vi "PLC_comm.vi"() -> ()   [LabVIEW 2017]
uses:
  <vilib>/DATA AHEAD/SP7/typedefs/PLC Type.ctl
  <vilib>/Utility/error.llb/DialogType.ctl
  <vilib>/addons/database/Connection.llb/DB Tools Open Connec (String).vi
  <vilib>/DATA AHEAD/SP7/functions/write/write Dint array.vi
  Global/Global 1.vi
  Global/DATA LOG.vi
  <vilib>/DATA AHEAD/SP7/functions/write/writeString.vi
  <vilib>/DATA AHEAD/SP7/functions/read/read Dint array.vi
  <vilib>/DATA AHEAD/SP7/functions/read/read real array.vi
  <vilib>/DATA AHEAD/SP7/functions/read/read String.vi
  <vilib>/addons/database/NI_Database_API.lvlib
  <vilib>/DATA AHEAD/SP7/SP7.lvlib
panel:
  out "error out 4":errorcluster
  out "error out 3":errorcluster
  out "error out 2":errorcluster
  out "IP1 8":string
  out "PLC 8":bool
  out "IP1 7":string
  out "PLC 7":bool
  out "IP1 6":string
  out "PLC 6":bool
  out "IP1 5":string
  out "PLC 5":bool
  out "PLC 4":bool
  out "PLC 3":bool
  out "PLC 2":bool
  out "PLC 1":bool
  out "IP1 4":string
  out "IP1 3":string
  out "IP1 2":string
  out "IP1":string
  in  "stop":bool
  out "error out":errorcluster
  in  "error in (no error)":errorcluster
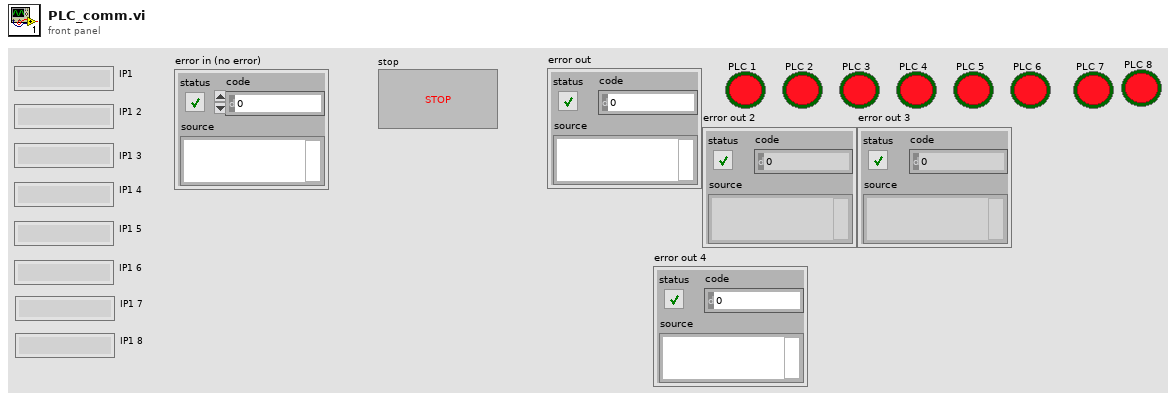
[diagram p1: front panel]
types:
  T1 = typedef "SP7.lvlib/PLC Type.ctl" = enum16{"S7 200", "S7 300/400", "S7 1200", "S7 1500", "LOGO!8"}
  T2 = typedef "DialogType.ctl" = u16
  T3 = typedef "NI_Database_API.lvlib/Conn ObjectReference.ctl" = refnum<k1>
  T4 = typedef "SP7.lvlib/S7 Connection.ctl" = cluster{"TCP Connection Ref":refnum<k5>, "IP address":string, "timeout ms":i32, "Connected?":bool, "PLC Type":T1, "Rack S7 400":u8, "Slot S7 400":u8, "PDU Size":u16, "connection semaphore":T5}
  T5 = typedef "Semaphore RefNum" = refnum<k1>
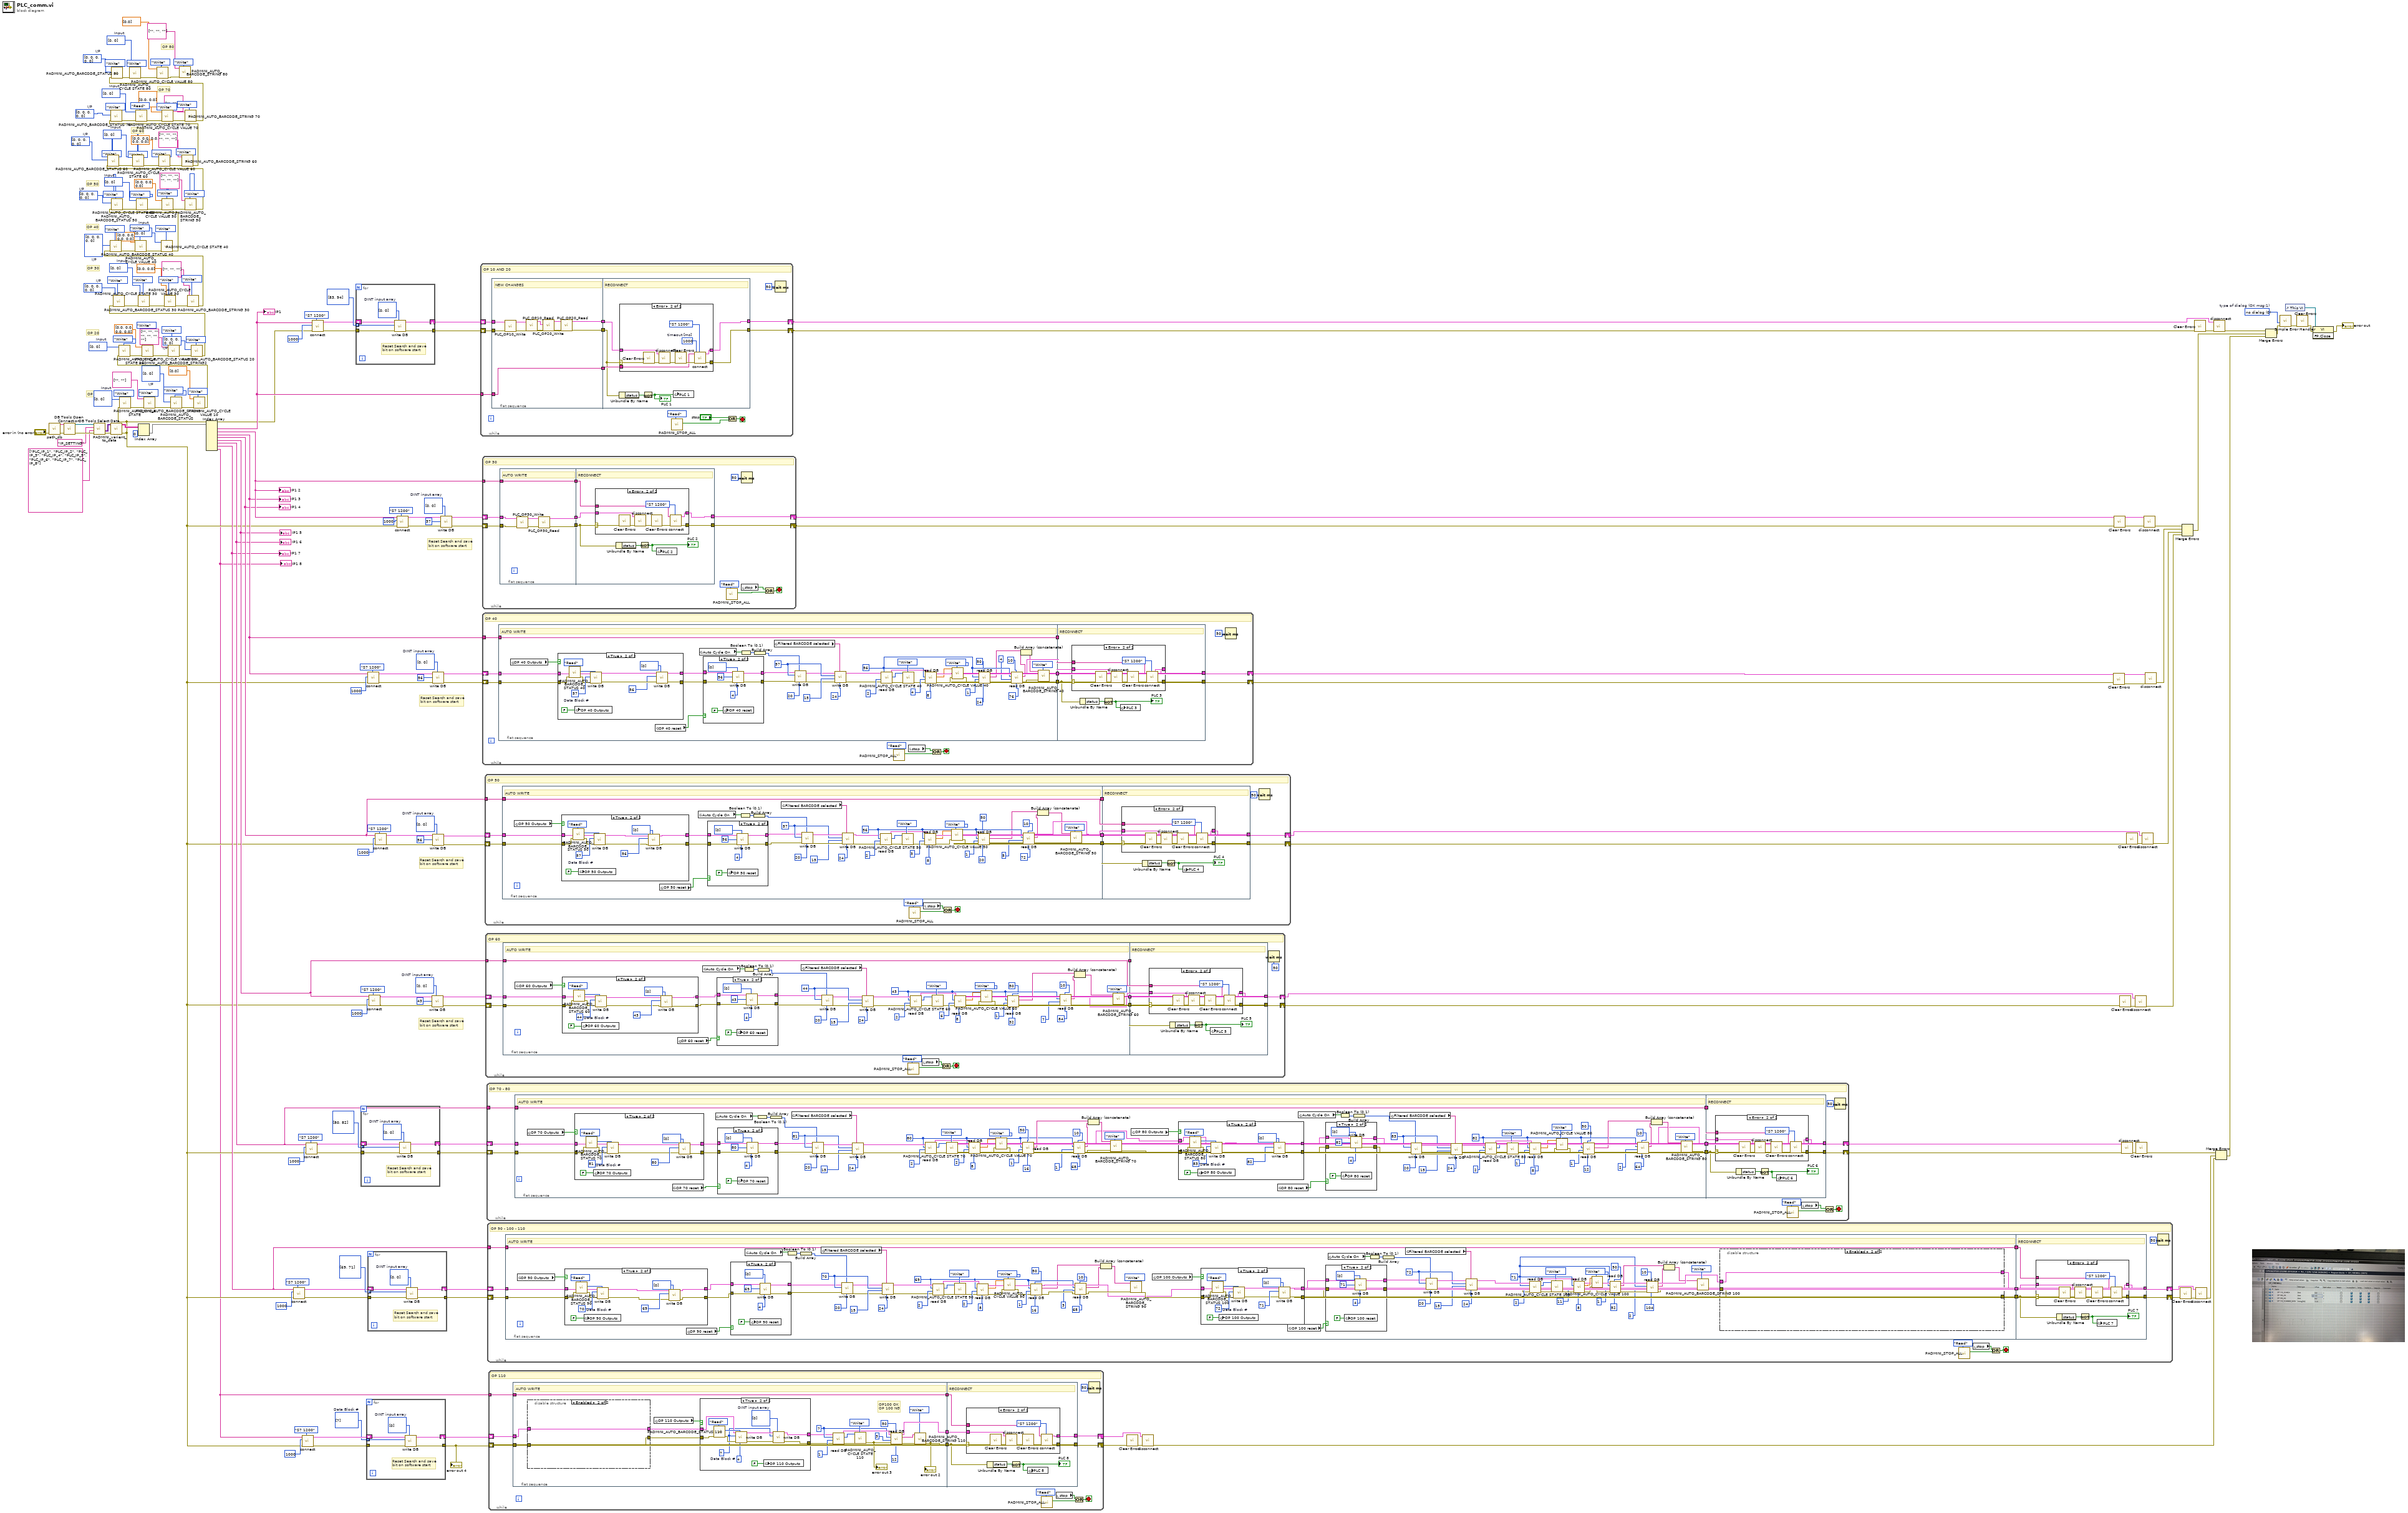
[diagram p0: block diagram]
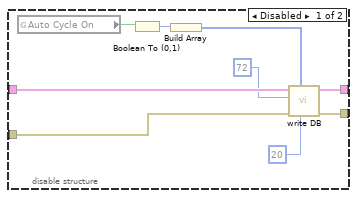
[diagram p2: hidden frame]
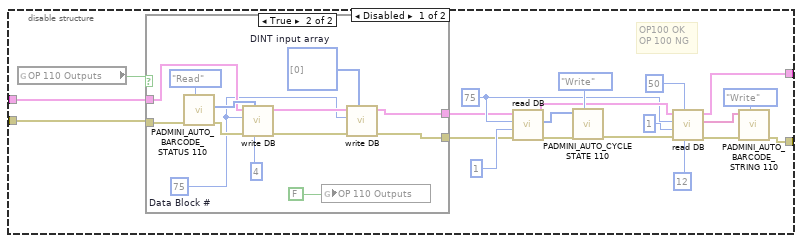
[diagram p5: hidden frame]
diagram:
  w6 = u16[] [7]  # Data Block #
  w28 = i32[] [0, 0]  # DINT input array
  w35 = i32[] [0, 0]  # DINT input array
  w40 = i32[] [0, 0]  # DINT input array
  w52 = i32[] [0, 0]  # DINT input array
  w53 = T2 0 items=["no dialog", "OK message", "continue or stop message", "OK message + warnings", "continue/stop + warnings"]  # type of dialog (OK msg:1)
  w55 = i32[] [0, 0, 0, 0, 0]  # I/P
  w56 = i32[] [0, 0]  # Input
  w58 = i32[] [0, 0]  # Input
  w59 = i32[] [0, 0]  # Input
  w61 = i32[] [0, 0]  # Input
  w57 = i32[] [0, 0, 0, 0, 0]  # I/P
  w60 = i32[] [0, 0, 0, 0, 0]  # I/P
  w62 = i32[] [0, 0, 0, 0, 0]  # I/P
  w63 = i32[] [0, 0, 0, 0, 0]  # I/P
  w64 = i32[] [0, 0]  # Input
  w65 = i32[] [0, 0]  # Input
  w66 = i32[] [0, 0, 0, 0, 0]  # I/P
  w67 = i32[] [0, 0, 0, 0, 0]  # I/P
  w68 = i32[] [0, 0]  # Input
  w69 = i32[] [0, 0]  # I/P
  w70 = i32[] [0, 0]  # Input
  # "Reset Search and save \nbit on software start"
  # "Reset Search and save \nbit on software start"
  # "Reset Search and save \nbit on software start"
  # "Reset Search and save \nbit on software start"
  # "OP 80"
  # "OP 70"
  # "OP 60"
  # "OP 50"
  # "OP 40"
  # "OP 30"
  # "OP 20"
  # "OP 10"
  n1 = call "path_db.vi"("error in"="error in (no error)") -> ("error out"=w208:errorcluster, "resulting string"=w213:string)  [unwired: 9 in]
  n2 = call-poly <vilib>:"DB Tools Open Connection.vi"("error in (no error)"=w208, "connection information"=w213) -> ("error out"=w212:errorcluster, "connection reference"=w211:T3)  [unwired: 6 in]
  n3 = call <vilib>:"DB Tools Select Data.vi"("error in (no error)"=w212, "columns"=string[] ["PLC_IP_1", "PLC_IP_2", "PLC_IP_3", "PLC_IP_4", "PLC_IP_5", "PLC_IP_6", "PLC_IP_7", "PLC_IP_8"], "table"="IP_SETTING", "connection reference"=w211) -> ("error out"=w210:errorcluster, "data"=w209:variant[][])  [unwired: 2 in, 1 out]
  n4 = call "PADMINI_varient_to_data.vi"("error in (no error)"=w210, "data"=w209) -> ("error out"=w7:errorcluster, "Array"=w204:string[][])  [unwired: 8 in]
  n5 = call "PADMINI_AUTO_CYCLE STATE.vi"("Enum"=enum16{"Read", "Write"}."Write", "error in (no error)"=w7, "Input"=w70) -> ("error out"=w192:errorcluster)  [unwired: 7 in, 1 out]
  n6 = Index Array(array=w204, index (row)=0) -> (element=w203:string[])  [unwired: 1 in]
  n7 = call "PADMINI_AUTO_BARCODE_STRING.vi"("Enum"=enum16{"Read", "Write"}."Write", "error in (no error)"=w192, "Input"=string[] ["", ""]) -> ("error out"=w189:errorcluster)  [unwired: 7 in, 1 out]
  n8 = call "PADMINI_AUTO_BARCODE_STATUS.vi"("Enum"=enum16{"Read", "Write"}."Write", "error in (no error)"=w189, "I/P"=w69) -> ("error out"=w187:errorcluster)  [unwired: 7 in, 1 out]
  n9 = call "PADMINI_AUTO_CYCLE VALUE 10.vi"("Enum"=enum16{"Read", "Write"}."Write", "error in (no error)"=w187, "Input"=dbl[] [0.0]) -> ("error out"=w181:errorcluster)  [unwired: 7 in, 1 out]
  n10 = call "PADMINI_AUTO_CYCLE STATE 20.vi"("Enum"=enum16{"Read", "Write"}."Write", "error in (no error)"=w181, "Input"=w56) -> ("error out"=w179:errorcluster)  [unwired: 7 in, 1 out]
  n11 = call "PADMINI_AUTO_CYCLE VALUE 20.vi"("Enum"=enum16{"Read", "Write"}."Write", "error in (no error)"=w179, "Input"=dbl[] [0.0, 0.0, 0.0, 0.0]) -> ("error out"=w175:errorcluster)  [unwired: 7 in, 1 out]
  n12 = call "PADMINI_AUTO_BARCODE_STRING2.vi"("Enum"=enum16{"Read", "Write"}."Write", "error in (no error)"=w175, "Input"=string[] ["", "", "", "", "", "", ""]) -> ("error out"=w173:errorcluster)  [unwired: 7 in, 1 out]
  n13 = call "PADMINI_AUTO_BARCODE_STATUS 20.vi"("Enum"=enum16{"Read", "Write"}."Write", "error in (no error)"=w173, "I/P"=w55) -> ("error out"=w169:errorcluster)  [unwired: 7 in, 1 out]
  n14 = call "PADMINI_AUTO_BARCODE_STATUS 30.vi"("Enum"=enum16{"Read", "Write"}."Write", "error in (no error)"=w169, "I/P"=w57) -> ("error out"=w166:errorcluster)  [unwired: 7 in, 1 out]
  n15 = call "PADMINI_AUTO_CYCLE STATE 30.vi"("Enum"=enum16{"Read", "Write"}."Write", "error in (no error)"=w166, "Input"=w58) -> ("error out"=w165:errorcluster)  [unwired: 7 in, 1 out]
  n16 = call "PADMINI_AUTO_CYCLE VALUE 30.vi"("Enum"=enum16{"Read", "Write"}."Write", "error in (no error)"=w165, "Input"=dbl[] [0.0, 0.0]) -> ("error out"=w162:errorcluster)  [unwired: 7 in, 1 out]
  n17 = call "PADMINI_AUTO_BARCODE_STRING 30.vi"("Enum"=enum16{"Read", "Write"}."Write", "error in (no error)"=w162, "Input"=string[] ["", "", ""]) -> ("error out"=w143:errorcluster)  [unwired: 7 in, 1 out]
  n18 = call "PADMINI_AUTO_BARCODE_STATUS 40.vi"("Enum"=enum16{"Read", "Write"}."Write", "error in (no error)"=w143, "I/P"=w60) -> ("error out"=w142:errorcluster)  [unwired: 7 in, 1 out]
  n19 = call "PADMINI_AUTO_CYCLE VALUE 40.vi"("Enum"=enum16{"Read", "Write"}."Write", "error in (no error)"=w142, "Input"=dbl[] [0.0, 0.0, 0.0, 0.0]) -> ("error out"=w141:errorcluster)  [unwired: 7 in, 1 out]
  n20 = call "PADMINI_AUTO_CYCLE STATE 40.vi"("Enum"=enum16{"Read", "Write"}."Write", "error in (no error)"=w141, "Input"=w59) -> ("error out"=w140:errorcluster)  [unwired: 7 in, 1 out]
  n21 = call "PADMINI_AUTO_BARCODE_STATUS 50.vi"("Enum"=enum16{"Read", "Write"}."Write", "error in (no error)"=w140, "I/P"=w62) -> ("error out"=w127:errorcluster)  [unwired: 7 in, 1 out]
  n22 = call "PADMINI_AUTO_CYCLE STATE 50.vi"("Enum"=enum16{"Read", "Write"}."Write", "error in (no error)"=w127, "Input"=w61) -> ("error out"=w131:errorcluster)  [unwired: 7 in, 1 out]
  n23 = call "PADMINI_AUTO_CYCLE VALUE 50.vi"("Enum"=enum16{"Read", "Write"}."Write", "error in (no error)"=w131, "Input"=dbl[] [0.0, 0.0, 0.0]) -> ("error out"=w128:errorcluster)  [unwired: 7 in, 1 out]
  n24 = call "PADMINI_AUTO_BARCODE_STRING 50.vi"("Enum"=enum16{"Read", "Write"}."Write", "error in (no error)"=w128, "Input"=string[] ["", "", "", "", "", ""]) -> ("error out"=w106:errorcluster)  [unwired: 7 in, 1 out]
  n25 = call "PADMINI_AUTO_BARCODE_STATUS 60.vi"("Enum"=enum16{"Read", "Write"}."Write", "error in (no error)"=w106, "I/P"=w63) -> ("error out"=w110:errorcluster)  [unwired: 7 in, 1 out]
  n26 = call "PADMINI_AUTO_CYCLE STATE 60.vi"("Enum"=enum16{"Read", "Write"}."Write", "error in (no error)"=w110, "Input"=w64) -> ("error out"=w112:errorcluster)  [unwired: 7 in, 1 out]
  n27 = call "PADMINI_AUTO_CYCLE VALUE 60.vi"("Enum"=enum16{"Read", "Write"}."Write", "error in (no error)"=w112, "Input"=dbl[] [0.0, 0.0, 0.0, 0.0, 0.0]) -> ("error out"=w115:errorcluster)  [unwired: 7 in, 1 out]
  n28 = call "PADMINI_AUTO_BARCODE_STRING 60.vi"("Enum"=enum16{"Read", "Write"}."Write", "error in (no error)"=w115, "Input"=string[] ["", "", "", "", "", ""]) -> ("error out"=w84:errorcluster)  [unwired: 7 in, 1 out]
  n29 = call "PADMINI_AUTO_BARCODE_STATUS 70.vi"("Enum"=enum16{"Read", "Write"}."Write", "error in (no error)"=w84, "I/P"=w66) -> ("error out"=w87:errorcluster)  [unwired: 7 in, 1 out]
  n30 = call "PADMINI_AUTO_CYCLE STATE 70.vi"("Enum"=enum16{"Read", "Write"}."Read", "error in (no error)"=w87, "Input"=w65) -> ("error out"=w99:errorcluster)  [unwired: 7 in, 1 out]
  n31 = call "PADMINI_AUTO_CYCLE VALUE 70.vi"("Enum"=enum16{"Read", "Write"}."Write", "error in (no error)"=w99, "Input"=dbl[] [0.0, 0.0]) -> ("error out"=w96:errorcluster)  [unwired: 7 in, 1 out]
  n32 = call "PADMINI_AUTO_BARCODE_STRING 70.vi"("Enum"=enum16{"Read", "Write"}."Write", "error in (no error)"=w96, "Input"=string[] ["", ""]) -> ("error out"=w81:errorcluster)  [unwired: 7 in, 1 out]
  n33 = call "PADMINI_AUTO_BARCODE_STATUS 80.vi"("Enum"=enum16{"Read", "Write"}."Write", "error in (no error)"=w81, "I/P"=w67) -> ("error out"=w88:errorcluster)  [unwired: 7 in, 1 out]
  n34 = call "PADMINI_AUTO_CYCLE STATE 80.vi"("Enum"=enum16{"Read", "Write"}."Write", "error in (no error)"=w88, "Input"=w68) -> ("error out"=w92:errorcluster)  [unwired: 7 in, 1 out]
  n35 = call "PADMINI_AUTO_CYCLE VALUE 80.vi"("Enum"=enum16{"Read", "Write"}."Write", "error in (no error)"=w92, "Input"=sgl[] [0.0]) -> ("error out"=w95:errorcluster)  [unwired: 7 in, 1 out]
  n36 = call "PADMINI_AUTO_BARCODE_STRING 80.vi"("Enum"=enum16{"Read", "Write"}."Write", "error in (no error)"=w95, "Input"=string[] ["", "", ""]) -> ()  [unwired: 7 in, 2 out]
  n37 = Index Array(array=w203) -> (element #1=w156:string, element #2=w157:string, element #3=w153:string, element #4=w133:string, element #5=w118:string, element #6=w78:string, element #7=w77:string, element #8=w5:string)  [unwired: 8 in]
  "IP1" <- w156
  "IP1 2" <- w157
  "IP1 3" <- w153
  "IP1 4" <- w133
  "IP1 5" <- w118
  "IP1 6" <- w78
  "IP1 7" <- w77
  "IP1 8" <- w5
  n38 = call <vilib>:"connect.vi"("PLC Type"=PLC_Type."S7 1200" ("PLC Type 2"), "error in (no error)"=w7, "timeout [ms]"=1000 ("timeout [ms] 2"), "IP address"=w77) -> ("error out"=w15:errorcluster, "S7 Connection out"=w14:T4)  [unwired: 6 in]
  n39 = call <vilib>:"connect.vi"("PLC Type"=PLC_Type."S7 1200" ("PLC Type 2"), "error in (no error)"=w7, "timeout [ms]"=1000 ("timeout [ms] 2"), "IP address"=w5) -> ("error out"=w9:errorcluster, "S7 Connection out"=w8:T4)  [unwired: 6 in]
  n40 = call <vilib>:"connect.vi"("PLC Type"=PLC_Type."S7 1200" ("PLC Type 2"), "error in (no error)"=w7, "timeout [ms]"=1000 ("timeout [ms] 2"), "IP address"=w78) -> ("error out"=w19:errorcluster, "S7 Connection out"=w20:T4)  [unwired: 6 in]
  n41 = call <vilib>:"connect.vi"("PLC Type"=PLC_Type."S7 1200" ("PLC Type 2"), "error in (no error)"=w7, "timeout [ms]"=1000, "IP address"=w156) -> ("error out"=w43:errorcluster, "S7 Connection out"=w42:T4)  [unwired: 6 in]
  n42 = for {
    tunnel: u16[] [83, 94] ("Data Block #") -> [w219] mode=indexing
    shift-right: [w217] -> w45
    shift-left: w42 -> [w214]
    tunnel: w43 -> [w215]
    tunnel: [w216] -> w44
    w218 = i32[] [0, 0]  # DINT input array
    # "Reset Search and save \nbit on software start"
    n43 = call-poly <vilib>:"write DB.vi"("DINT input array"=w218, "error in (no error)"=w215, "Data Block #"=w219, "S7 Connection in"=w214) -> ("error out"=w216:errorcluster, "S7 Connection out"=w217:T4)  [unwired: 4 in, 2 out]
  }
  n44 = for {
    tunnel: u16[] [80, 82] ("Data Block #") -> [w225] mode=indexing
    shift-right: [w223] -> w21
    shift-left: w20 -> [w220]
    tunnel: w19 -> [w221]
    tunnel: [w222] -> w22
    w224 = i32[] [0, 0]  # DINT input array
    # "Reset Search and save \nbit on software start"
    n45 = call-poly <vilib>:"write DB.vi"("DINT input array"=w224, "error in (no error)"=w221, "Data Block #"=w225, "S7 Connection in"=w220) -> ("error out"=w222:errorcluster, "S7 Connection out"=w223:T4)  [unwired: 4 in, 2 out]
  }
  n46 = for {
    tunnel: w6 -> [w231] mode=indexing
    shift-right: [w229] -> w12
    shift-left: w8 -> [w226]
    tunnel: w9 -> [w227]
    tunnel: [w228] -> w13
    w230 = i32[] [0]  # DINT input array
    # "Reset Search and save \nbit on software start"
    n47 = call-poly <vilib>:"write DB.vi"("DINT input array"=w230, "error in (no error)"=w227, "Data Block #"=w231, "S7 Connection in"=w226) -> ("error out"=w228:errorcluster, "S7 Connection out"=w229:T4)  [unwired: 4 in, 2 out]
  }
  "error out 4" <- w13
  n48 = call <vilib>:"connect.vi"("PLC Type"=PLC_Type."S7 1200" ("PLC Type 2"), "error in (no error)"=w7, "timeout [ms]"=1000 ("timeout [ms] 2"), "IP address"=w153) -> ("error out"=w37:errorcluster, "S7 Connection out"=w36:T4)  [unwired: 6 in]
  n49 = for {
    tunnel: u16[] [69, 71] ("Data Block #") -> [w237] mode=indexing
    shift-right: [w235] -> w17
    shift-left: w14 -> [w232]
    tunnel: w15 -> [w233]
    tunnel: [w234] -> w16
    w236 = i32[] [0, 0]  # DINT input array
    # "Reset Search and save \nbit on software start"
    n50 = call-poly <vilib>:"write DB.vi"("DINT input array"=w236, "error in (no error)"=w233, "Data Block #"=w237, "S7 Connection in"=w232) -> ("error out"=w234:errorcluster, "S7 Connection out"=w235:T4)  [unwired: 4 in, 2 out]
  }
  n51 = call <vilib>:"connect.vi"("PLC Type"=PLC_Type."S7 1200" ("PLC Type 2"), "error in (no error)"=w7, "timeout [ms]"=1000 ("timeout [ms] 2"), "IP address"=w118) -> ("error out"=w24:errorcluster, "S7 Connection out"=w25:T4)  [unwired: 6 in]
  n52 = call <vilib>:"connect.vi"("PLC Type"=PLC_Type."S7 1200" ("PLC Type 2"), "error in (no error)"=w7, "timeout [ms]"=1000 ("timeout [ms] 2"), "IP address"=w133) -> ("error out"=w31:errorcluster, "S7 Connection out"=w30:T4)  [unwired: 6 in]
  n53 = call <vilib>:"connect.vi"("PLC Type"=PLC_Type."S7 1200" ("PLC Type 2"), "error in (no error)"=w7, "timeout [ms]"=1000 ("timeout [ms] 2"), "IP address"=w157) -> ("error out"=w49:errorcluster, "S7 Connection out"=w50:T4)  [unwired: 6 in]
  n54 = call-poly <vilib>:"write DB.vi"("DINT input array"=w28, "error in (no error)"=w24, "Data Block #"=u16 43, "S7 Connection in"=w25) -> ("error out"=w27:errorcluster, "S7 Connection out"=w26:T4)  [unwired: 4 in, 2 out]
  n55 = call-poly <vilib>:"write DB.vi"("DINT input array"=w35, "error in (no error)"=w31, "Data Block #"=u16 56, "S7 Connection in"=w30) -> ("error out"=w32:errorcluster, "S7 Connection out"=w33:T4)  [unwired: 4 in, 2 out]
  n56 = call-poly <vilib>:"write DB.vi"("DINT input array"=w40, "error in (no error)"=w37, "Data Block #"=u16 56, "S7 Connection in"=w36) -> ("error out"=w39:errorcluster, "S7 Connection out"=w38:T4)  [unwired: 4 in, 2 out]
  n57 = call-poly <vilib>:"write DB.vi"("DINT input array"=w52, "error in (no error)"=w49, "Data Block #"=u16 37, "S7 Connection in"=w50) -> ("error out"=w48:errorcluster, "S7 Connection out"=w47:T4)  [unwired: 4 in, 2 out]
  n58 = while {
    shift-right: [w240] -> w184
    shift-left: w45 -> [w250]
    shift-right: [w248] -> w197
    shift-left: w44 -> [w249]
    tunnel: w156 -> [w238]
    stop <- w243 stop-if-true
    # "OP 10 AND 20"
    n59 = flat-sequence {
      tunnel: [w253] -> w242
      tunnel: [w259] -> w241
      tunnel: w249 -> [w260]
      tunnel: w250 -> [w261]
      tunnel: [w258] -> w239
      tunnel: w238 -> [w258]
      tunnel: [w265] -> w248
      tunnel: [w264] -> w240
      tunnel: w242 -> [w266]
      tunnel: w241 -> [w262]
      tunnel: w239 -> [w263]
      frame #0 {
        # "NEW CHANGES"
        n60 = call "PLC_OP10_Write.vi"("error in (no error)"=w260, "S7 Connection in"=w261) -> ("error out"=w256:errorcluster, "S7 Connection out"=w257:T4)  [unwired: 8 in]
        n61 = call "PLC_OP10_Read.vi"("error in (no error)"=w256, "S7 Connection in"=w257) -> ("error out"=w255:errorcluster, "S7 Connection out"=w254:T4)  [unwired: 8 in]
        n62 = call "PLC_OP20_Write.vi"("error in (no error)"=w255, "S7 Connection in"=w254) -> ("error out"=w251:errorcluster, "S7 Connection out"=w252:T4)  [unwired: 8 in]
        n63 = call "PLC_OP20_Read.vi"("error in (no error)"=w251, "S7 Connection in"=w252) -> ("error out"=w259:errorcluster, "S7 Connection out 2"=w253:T4)  [unwired: 8 in]
      }
      frame #1 {
        # "RECONNECT"
        n64 = Unbundle By Name(w262) -> ("status"=w268:bool)
        n65 = case shown="Error" w262 {
          selector: w262 -> [w270 w279]
          tunnel: [w269 w276] -> w264
          tunnel: [w270 w277] -> w265
          tunnel: w266 -> [w269 w273]
          tunnel: w263 -> [_ w272]
          frame No Error {
          }
          frame Error {
            w271 = 1000  # timeout [ms]
            n66 = call <vilib>:"Clear Errors.vi"("error in (no error)"=w279) -> ("error out"=w280:errorcluster)  [unwired: 5 in, 1 out]
            n67 = call <vilib>:"disconnect.vi"("error in (no error)"=w280, "S7 Connection in"=w273) -> ("error out"=w278:errorcluster)  [unwired: 8 in, 1 out]
            n68 = call <vilib>:"Clear Errors.vi"("error in (no error)"=w278) -> ("error out"=w275:errorcluster)  [unwired: 5 in, 1 out]
            n69 = call <vilib>:"connect.vi"("PLC Type"=PLC_Type."S7 1200" ("PLC Type 2"), "error in (no error)"=w275, "timeout [ms]"=w271, "IP address"=w272) -> ("error out"=w277:errorcluster, "S7 Connection out"=w276:T4)  [unwired: 6 in]
          }
        }
        n70 = Not(x=w268) -> (.not. x?=w267:bool)
        "PLC 1" <- w267
        n71 = global write "Global 1.vi" "PLC 1"(w267) -> ()
      }
    }
    n72 = call "PADMINI_STOP_ALL.vi"("Enum"=enum16{"Read", "Write"}."Read") -> ("Boolean 2"=w245:bool)  [unwired: 9 in, 1 out]
    n73 = Or(x="stop", y=w245) -> (x .or. y?=w243:bool)
    n74 = Wait (ms)(milliseconds to wait=u32 50) -> ()  [unwired: 1 out]
  }
  n75 = while {
    shift-right: [w283] -> w159
    shift-left: w47 -> [w293]
    shift-right: [w291] -> w158
    shift-left: w48 -> [w292]
    tunnel: w157 -> [w282]
    stop <- w285 stop-if-true
    # "OP 30"
    n76 = flat-sequence {
      tunnel: [w296] -> w289
      tunnel: [w298] -> w284
      tunnel: w292 -> [w300]
      tunnel: w293 -> [w299]
      tunnel: w282 -> [w297]
      tunnel: [w297] -> w281
      tunnel: [w303] -> w291
      tunnel: [w302] -> w283
      tunnel: w289 -> [w305]
      tunnel: w284 -> [w304]
      tunnel: w281 -> [w301]
      frame #0 {
        # "AUTO WRITE"
        n77 = call "PLC_OP30_Write.vi"("error in (no error)"=w300, "S7 Connection in"=w299) -> ("error out"=w294:errorcluster, "S7 Connection out"=w295:T4)  [unwired: 8 in]
        n78 = call "PLC_OP30_Read.vi"("error in (no error)"=w294, "S7 Connection in"=w295) -> ("error out"=w298:errorcluster, "S7 Connection out 2"=w296:T4)  [unwired: 8 in]
      }
      frame #1 {
        # "RECONNECT"
        n79 = case shown="Error" w304 {
          selector: w304 -> [w309 w317]
          tunnel: [w308 w314] -> w302
          tunnel: [w309 w315] -> w303
          tunnel: w305 -> [w308 w311]
          tunnel: w301 -> [_ w310]
          frame No Error {
          }
          frame Error {
            n80 = call <vilib>:"Clear Errors.vi"("error in (no error)"=w317) -> ("error out"=w318:errorcluster)  [unwired: 5 in, 1 out]
            n81 = call <vilib>:"disconnect.vi"("error in (no error)"=w318, "S7 Connection in"=w311) -> ("error out"=w316:errorcluster)  [unwired: 8 in, 1 out]
            n82 = call <vilib>:"Clear Errors.vi"("error in (no error)"=w316) -> ("error out"=w313:errorcluster)  [unwired: 5 in, 1 out]
            n83 = call <vilib>:"connect.vi"("PLC Type"=PLC_Type."S7 1200" ("PLC Type 2"), "error in (no error)"=w313, "IP address"=w310) -> ("error out"=w315:errorcluster, "S7 Connection out"=w314:T4)  [unwired: 7 in]
          }
        }
        n84 = Unbundle By Name(w304) -> ("status"=w307:bool)
        n85 = Not(x=w307) -> (.not. x?=w306:bool)
        "PLC 2" <- w306
        n86 = global write "Global 1.vi" "PLC 2"(w306) -> ()
      }
    }
    n87 = call "PADMINI_STOP_ALL.vi"("Enum"=enum16{"Read", "Write"}."Read") -> ("Boolean 2"=w287:bool)  [unwired: 9 in, 1 out]
    n88 = Wait (ms)(milliseconds to wait=u32 50) -> ()  [unwired: 1 out]
    n89 = local read "stop"() -> (w286:bool)
    n90 = Or(x=w286, y=w287) -> (x .or. y?=w285:bool)
  }
  n91 = while {
    shift-right: [w321] -> w150
    shift-left: w38 -> [w331]
    shift-right: [w329] -> w151
    shift-left: w39 -> [w330]
    tunnel: w153 -> [w320]
    stop <- w323 stop-if-true
    # "OP 40"
    n92 = flat-sequence {
      tunnel: [w343] -> w327
      tunnel: [w362] -> w322
      tunnel: w330 -> [w381]
      tunnel: w331 -> [w380]
      tunnel: w320 -> [w361]
      tunnel: [w361] -> w319
      tunnel: [w409] -> w329
      tunnel: [w408] -> w321
      tunnel: w327 -> [w411]
      tunnel: w322 -> [w410]
      tunnel: w319 -> [w407]
      frame #0 {
        w354 = u16 57 ("Data Block #")
        w342 = u16 56 ("Data Block #")
        # "AUTO WRITE"
        n93 = global read "DATA LOG.vi" "OP 40 Outputs"() -> (w379:bool)
        n94 = case shown="True" w379 {
          tunnel: w380 -> [w392 w405]
          tunnel: [w393 w397] -> w359
          tunnel: [w392 w399] -> w360
          tunnel: w381 -> [w393 w402]
          frame False {
          }
          frame True {
            w406 = u16 57  # Data Block #
            n95 = call "PADMINI_AUTO_BARCODE_STATUS 40.vi"("Enum"=enum16{"Read", "Write"}."Read", "error in (no error)"=w402) -> ("error out"=w401:errorcluster, "O/P"=w403:i32[])  [unwired: 8 in]
            n96 = global write "DATA LOG.vi" "OP 40 Outputs"(FALSE) -> ()
            n97 = call-poly <vilib>:"write DB.vi"("DINT input array"=w403, "error in (no error)"=w401, "Data Block #"=w406, "S7 Connection in"=w405) -> ("error out"=w396:errorcluster, "S7 Connection out"=w398:T4)  [unwired: 4 in, 2 out]
            n98 = call-poly <vilib>:"write DB.vi"("DINT input array"=i32[] [0], "error in (no error)"=w396, "Data Block #"=u16 56, "S7 Connection in"=w398) -> ("error out"=w397:errorcluster, "S7 Connection out"=w399:T4)  [unwired: 4 in, 2 out]
          }
        }
        n99 = global read "DATA LOG.vi" "OP 40 reset"() -> (w358:bool)
        n100 = global read "DATA LOG.vi" "Auto Cycle On"() -> (w334:bool)
        n101 = case shown="True" w358 {
          tunnel: w359 -> [w382 w391]
          tunnel: [w382 w390] -> w347
          tunnel: w360 -> [w383 w389]
          tunnel: [w383 w388] -> w348
          frame False {
          }
          frame True {
            n102 = global write "DATA LOG.vi" "OP 40 reset"(FALSE) -> ()
            n103 = call-poly <vilib>:"write DB.vi"("Item offset [byte]"=u16 4 ("Data Block #"), "DINT input array"=i32[] [0], "error in (no error)"=w391, "Data Block #"=u16 56, "S7 Connection in"=w389) -> ("error out"=w390:errorcluster, "S7 Connection out"=w388:T4)  [unwired: 3 in, 2 out]
          }
        }
        n104 = Boolean To (0,1)(Boolean=w334) -> (0, 1=w333:i16)
        n105 = Build Array(w333) -> (w332:i16[])
        n106 = global read "Global 1.vi" "Filtered BARCODE selected"() -> (w357:string[])
        n107 = call-poly <vilib>:"write DB.vi"("Item offset [byte]"=u32 20, "DINT input array"=w332, "error in (no error)"=w347, "Data Block #"=w354, "S7 Connection in"=w348) -> ("error out"=w352:errorcluster, "S7 Connection out"=w351:T4)  [unwired: 3 in, 2 out]
        n108 = call-poly <vilib>:"write DB.vi"("Item offset [byte]"=u32 24, "Input STRINGS"=w357, "error in (no error)"=w352, "String length reserved in DB (default=254)"=u16 15, "Data Block #"=w354, "S7 Connection in"=w351) -> ("error out"=w349:errorcluster, "S7 Connection out"=w350:T4)  [unwired: 2 in, 2 out]
        n109 = call-poly <vilib>:"read DB.vi"("error in (no error)"=w349, "items #"=u16 2 ("Items # [byte]"), "Data Block #"=w342, "S7 Connection in"=w350) -> ("error out"=w377:errorcluster, "DINT result array"=w375:i32[], "S7 Connection out"=w372:T4)  [unwired: 5 in]
        n110 = call "PADMINI_AUTO_CYCLE STATE 40.vi"("Enum"=enum16{"Read", "Write"}."Write", "error in (no error)"=w377, "Input"=w375) -> ("error out"=w373:errorcluster)  [unwired: 7 in, 1 out]
        n111 = call-poly <vilib>:"read DB.vi"("Item offset [byte]"=u32 8, "error in (no error)"=w373, "items #"=u16 4 ("Items # [byte]"), "Data Block #"=w342, "S7 Connection in"=w372) -> ("error out"=w365:errorcluster, "REAL result array"=w363:sgl[], "S7 Connection out"=w371:T4)  [unwired: 4 in]
        n112 = call "PADMINI_AUTO_CYCLE VALUE 40.vi"("Enum"=enum16{"Read", "Write"}."Write", "error in (no error)"=w365, "Input"=w363) -> ("error out"=w364:errorcluster)  [unwired: 7 in, 1 out]
        n113 = call-poly <vilib>:"read DB.vi"("Item offset [byte]"=u32 24, "String length reserved in DB (default=254)"=u16 50, "error in (no error)"=w364, "items #"=u16 1 ("Items # [byte]"), "Data Block #"=w342, "S7 Connection in"=w371) -> ("error out"=w346:errorcluster, "STRING result Array"=w337:string[], "S7 Connection out"=w344:T4)  [unwired: 2 in, 1 out]
        n114 = call-poly <vilib>:"read DB.vi"("Item offset [byte]"=u32 76, "String length reserved in DB (default=254)"=u16 10, "error in (no error)"=w346, "items #"=u16 4 ("Items # [byte]"), "Data Block #"=w342, "S7 Connection in"=w344) -> ("error out"=w345:errorcluster, "STRING result Array"=w336:string[], "S7 Connection out"=w343:T4)  [unwired: 2 in, 1 out]
        n115 = Build Array (concatenate)(w337, w336) -> (w335:string[])
        n116 = call "PADMINI_AUTO_BARCODE_STRING 40.vi"("Enum"=enum16{"Read", "Write"}."Write", "error in (no error)"=w345, "Input"=w335) -> ("error out"=w362:errorcluster)  [unwired: 7 in, 1 out]
      }
      frame #1 {
        # "RECONNECT"
        n117 = case shown="Error" w410 {
          selector: w410 -> [w415 w423]
          tunnel: [w414 w420] -> w408
          tunnel: [w415 w421] -> w409
          tunnel: w411 -> [w414 w417]
          tunnel: w407 -> [_ w416]
          frame No Error {
          }
          frame Error {
            n118 = call <vilib>:"Clear Errors.vi"("error in (no error)"=w423) -> ("error out"=w424:errorcluster)  [unwired: 5 in, 1 out]
            n119 = call <vilib>:"disconnect.vi"("error in (no error)"=w424, "S7 Connection in"=w417) -> ("error out"=w422:errorcluster)  [unwired: 8 in, 1 out]
            n120 = call <vilib>:"Clear Errors.vi"("error in (no error)"=w422) -> ("error out"=w419:errorcluster)  [unwired: 5 in, 1 out]
            n121 = call <vilib>:"connect.vi"("PLC Type"=PLC_Type."S7 1200" ("PLC Type 2"), "error in (no error)"=w419, "IP address"=w416) -> ("error out"=w421:errorcluster, "S7 Connection out"=w420:T4)  [unwired: 7 in]
          }
        }
        n122 = Unbundle By Name(w410) -> ("status"=w413:bool)
        n123 = Not(x=w413) -> (.not. x?=w412:bool)
        "PLC 3" <- w412
        n124 = global write "Global 1.vi" "PLC 3"(w412) -> ()
      }
    }
    n125 = call "PADMINI_STOP_ALL.vi"("Enum"=enum16{"Read", "Write"}."Read") -> ("Boolean 2"=w325:bool)  [unwired: 9 in, 1 out]
    n126 = local read "stop"() -> (w324:bool)
    n127 = Or(x=w324, y=w325) -> (x .or. y?=w323:bool)
    n128 = Wait (ms)(milliseconds to wait=u32 50) -> ()  [unwired: 1 out]
  }
  n129 = while {
    shift-right: [w427] -> w138
    shift-left: w33 -> [w437]
    shift-right: [w435] -> w137
    shift-left: w32 -> [w436]
    tunnel: w133 -> [w426]
    stop <- w429 stop-if-true
    # "OP 50"
    n130 = flat-sequence {
      tunnel: [w458] -> w433
      tunnel: [w468] -> w428
      tunnel: w436 -> [w487]
      tunnel: w437 -> [w486]
      tunnel: w426 -> [w467]
      tunnel: [w467] -> w425
      tunnel: [w515] -> w435
      tunnel: [w514] -> w427
      tunnel: w433 -> [w517]
      tunnel: w428 -> [w516]
      tunnel: w425 -> [w513]
      frame #0 {
        w449 = u16 57 ("Data Block #")
        w457 = u16 56 ("Data Block #")
        # "AUTO WRITE"
        n131 = global read "DATA LOG.vi" "OP 50 Outputs"() -> (w485:bool)
        n132 = case shown="True" w485 {
          tunnel: w486 -> [w498 w511]
          tunnel: [w499 w500] -> w466
          tunnel: [w498 w503] -> w465
          tunnel: w487 -> [w499 w508]
          frame False {
          }
          frame True {
            w512 = u16 57  # Data Block #
            n133 = call "PADMINI_AUTO_BARCODE_STATUS 50.vi"("Enum"=enum16{"Read", "Write"}."Read", "error in (no error)"=w508) -> ("error out"=w507:errorcluster, "O/P"=w509:i32[])  [unwired: 8 in]
            n134 = global write "DATA LOG.vi" "OP 50 Outputs"(FALSE) -> ()
            n135 = call-poly <vilib>:"write DB.vi"("DINT input array"=w509, "error in (no error)"=w507, "Data Block #"=w512, "S7 Connection in"=w511) -> ("error out"=w501:errorcluster, "S7 Connection out"=w502:T4)  [unwired: 4 in, 2 out]
            n136 = call-poly <vilib>:"write DB.vi"("DINT input array"=i32[] [0] ("Data Byte"), "error in (no error)"=w501, "Data Block #"=u16 56, "S7 Connection in"=w502) -> ("error out"=w500:errorcluster, "S7 Connection out"=w503:T4)  [unwired: 4 in, 2 out]
          }
        }
        n137 = global read "DATA LOG.vi" "OP 50 reset"() -> (w464:bool)
        n138 = global read "DATA LOG.vi" "Auto Cycle On"() -> (w440:bool)
        n139 = case shown="True" w464 {
          tunnel: w466 -> [w488 w497]
          tunnel: [w488 w496] -> w442
          tunnel: w465 -> [w489 w495]
          tunnel: [w489 w494] -> w445
          frame False {
          }
          frame True {
            n140 = global write "DATA LOG.vi" "OP 50 reset"(FALSE) -> ()
            n141 = call-poly <vilib>:"write DB.vi"("Item offset [byte]"=u16 4 ("Data Block #"), "DINT input array"=i32[] [0], "error in (no error)"=w497, "Data Block #"=u16 56, "S7 Connection in"=w495) -> ("error out"=w496:errorcluster, "S7 Connection out"=w494:T4)  [unwired: 3 in, 2 out]
          }
        }
        n142 = Boolean To (0,1)(Boolean=w440) -> (0, 1=w439:i16)
        n143 = Build Array(w439) -> (w438:i16[])
        n144 = global read "Global 1.vi" "Filtered BARCODE selected"() -> (w446:string[])
        n145 = call-poly <vilib>:"write DB.vi"("Item offset [byte]"=u32 20, "DINT input array"=w438, "error in (no error)"=w442, "Data Block #"=w449, "S7 Connection in"=w445) -> ("error out"=w451:errorcluster, "S7 Connection out"=w452:T4)  [unwired: 3 in, 2 out]
        n146 = call-poly <vilib>:"write DB.vi"("Item offset [byte]"=u32 24, "Input STRINGS"=w446, "error in (no error)"=w451, "String length reserved in DB (default=254)"=u16 15, "Data Block #"=w449, "S7 Connection in"=w452) -> ("error out"=w443:errorcluster, "S7 Connection out"=w444:T4)  [unwired: 2 in, 2 out]
        n147 = call-poly <vilib>:"read DB.vi"("error in (no error)"=w443, "items #"=u16 2 ("Items # [byte]"), "Data Block #"=w457, "S7 Connection in"=w444) -> ("error out"=w483:errorcluster, "DINT result array"=w481:i32[], "S7 Connection out"=w478:T4)  [unwired: 5 in]
        n148 = call "PADMINI_AUTO_CYCLE STATE 50.vi"("Enum"=enum16{"Read", "Write"}."Write", "error in (no error)"=w483, "Input"=w481) -> ("error out"=w479:errorcluster)  [unwired: 7 in, 1 out]
        n149 = call-poly <vilib>:"read DB.vi"("Item offset [byte]"=u32 8, "error in (no error)"=w479, "items #"=u16 3 ("Items # [byte]"), "Data Block #"=w457, "S7 Connection in"=w478) -> ("error out"=w471:errorcluster, "REAL result array"=w469:sgl[], "S7 Connection out"=w477:T4)  [unwired: 4 in]
        n150 = call "PADMINI_AUTO_CYCLE VALUE 50.vi"("Enum"=enum16{"Read", "Write"}."Write", "error in (no error)"=w471, "Input"=w469) -> ("error out"=w470:errorcluster)  [unwired: 7 in, 1 out]
        n151 = call-poly <vilib>:"read DB.vi"("Item offset [byte]"=u32 20, "String length reserved in DB (default=254)"=u16 50, "error in (no error)"=w470, "items #"=u16 1 ("Items # [byte]"), "Data Block #"=w457, "S7 Connection in"=w477) -> ("error out"=w460:errorcluster, "STRING result Array"=w456:string[], "S7 Connection out"=w459:T4)  [unwired: 2 in, 1 out]
        n152 = call-poly <vilib>:"read DB.vi"("Item offset [byte]"=u32 72, "String length reserved in DB (default=254)"=u16 10, "error in (no error)"=w460, "items #"=u16 5 ("Items # [byte]"), "Data Block #"=w457, "S7 Connection in"=w459) -> ("error out"=w461:errorcluster, "STRING result Array"=w455:string[], "S7 Connection out"=w458:T4)  [unwired: 2 in, 1 out]
        n153 = Build Array (concatenate)(w456, w455) -> (w454:string[])
        n154 = call "PADMINI_AUTO_BARCODE_STRING 50.vi"("Enum"=enum16{"Read", "Write"}."Write", "error in (no error)"=w461, "Input"=w454) -> ("error out"=w468:errorcluster)  [unwired: 7 in, 1 out]
      }
      frame #1 {
        # "RECONNECT"
        n155 = case shown="Error" w516 {
          selector: w516 -> [w521 w529]
          tunnel: [w520 w526] -> w514
          tunnel: [w521 w527] -> w515
          tunnel: w517 -> [w520 w523]
          tunnel: w513 -> [_ w522]
          frame No Error {
          }
          frame Error {
            n156 = call <vilib>:"Clear Errors.vi"("error in (no error)"=w529) -> ("error out"=w530:errorcluster)  [unwired: 5 in, 1 out]
            n157 = call <vilib>:"disconnect.vi"("error in (no error)"=w530, "S7 Connection in"=w523) -> ("error out"=w528:errorcluster)  [unwired: 8 in, 1 out]
            n158 = call <vilib>:"Clear Errors.vi"("error in (no error)"=w528) -> ("error out"=w525:errorcluster)  [unwired: 5 in, 1 out]
            n159 = call <vilib>:"connect.vi"("PLC Type"=PLC_Type."S7 1200" ("PLC Type 2"), "error in (no error)"=w525, "IP address"=w522) -> ("error out"=w527:errorcluster, "S7 Connection out"=w526:T4)  [unwired: 7 in]
          }
        }
        n160 = Unbundle By Name(w516) -> ("status"=w519:bool)
        n161 = Not(x=w519) -> (.not. x?=w518:bool)
        "PLC 4" <- w518
        n162 = global write "Global 1.vi" "PLC 4"(w518) -> ()
      }
    }
    n163 = call "PADMINI_STOP_ALL.vi"("Enum"=enum16{"Read", "Write"}."Read") -> ("Boolean 2"=w431:bool)  [unwired: 9 in, 1 out]
    n164 = local read "stop"() -> (w430:bool)
    n165 = Or(x=w430, y=w431) -> (x .or. y?=w429:bool)
    n166 = Wait (ms)(milliseconds to wait=u32 50) -> ()  [unwired: 1 out]
  }
  n167 = while {
    shift-right: [w533] -> w119
    shift-left: w26 -> [w543]
    shift-right: [w541] -> w120
    shift-left: w27 -> [w542]
    tunnel: w118 -> [w532]
    stop <- w535 stop-if-true
    # "OP 60"
    n168 = flat-sequence {
      tunnel: [w552] -> w539
      tunnel: [w574] -> w534
      tunnel: w542 -> [w593]
      tunnel: w543 -> [w592]
      tunnel: w532 -> [w573]
      tunnel: [w573] -> w531
      tunnel: [w621] -> w541
      tunnel: [w620] -> w533
      tunnel: w539 -> [w623]
      tunnel: w534 -> [w622]
      tunnel: w531 -> [w619]
      frame #0 {
        w569 = u16 44 ("Data Block #")
        w549 = u16 43 ("Data Block #")
        # "AUTO WRITE"
        n169 = global read "DATA LOG.vi" "OP 60 Outputs"() -> (w591:bool)
        n170 = case shown="True" w591 {
          tunnel: w592 -> [w604 w617]
          tunnel: [w605 w606] -> w561
          tunnel: [w604 w609] -> w560
          tunnel: w593 -> [w605 w614]
          frame False {
          }
          frame True {
            w618 = u16 44  # Data Block #
            n171 = call "PADMINI_AUTO_BARCODE_STATUS 60.vi"("Enum"=enum16{"Read", "Write"}."Read", "error in (no error)"=w614) -> ("error out"=w613:errorcluster, "O/P"=w615:i32[])  [unwired: 8 in]
            n172 = global write "DATA LOG.vi" "OP 60 Outputs"(FALSE) -> ()
            n173 = call-poly <vilib>:"write DB.vi"("DINT input array"=w615, "error in (no error)"=w613, "Data Block #"=w618, "S7 Connection in"=w617) -> ("error out"=w607:errorcluster, "S7 Connection out"=w608:T4)  [unwired: 4 in, 2 out]
            n174 = call-poly <vilib>:"write DB.vi"("DINT input array"=i32[] [0] ("Data Byte"), "error in (no error)"=w607, "Data Block #"=u16 43, "S7 Connection in"=w608) -> ("error out"=w606:errorcluster, "S7 Connection out"=w609:T4)  [unwired: 4 in, 2 out]
          }
        }
        n175 = global read "DATA LOG.vi" "OP 60 reset"() -> (w559:bool)
        n176 = global read "DATA LOG.vi" "Auto Cycle On"() -> (w546:bool)
        n177 = case shown="True" w559 {
          tunnel: w561 -> [w594 w603]
          tunnel: [w594 w602] -> w562
          tunnel: w560 -> [w595 w601]
          tunnel: [w595 w600] -> w563
          frame False {
          }
          frame True {
            n178 = global write "DATA LOG.vi" "OP 60 reset"(FALSE) -> ()
            n179 = call-poly <vilib>:"write DB.vi"("Item offset [byte]"=u16 4 ("Data Block #"), "DINT input array"=i32[] [0], "error in (no error)"=w603, "Data Block #"=u16 43, "S7 Connection in"=w601) -> ("error out"=w602:errorcluster, "S7 Connection out"=w600:T4)  [unwired: 3 in, 2 out]
          }
        }
        n180 = Boolean To (0,1)(Boolean=w546) -> (0, 1=w545:i16)
        n181 = Build Array(w545) -> (w544:i16[])
        n182 = global read "Global 1.vi" "Filtered BARCODE selected"() -> (w572:string[])
        n183 = call-poly <vilib>:"write DB.vi"("Item offset [byte]"=u32 20, "DINT input array"=w544, "error in (no error)"=w562, "Data Block #"=w569, "S7 Connection in"=w563) -> ("error out"=w567:errorcluster, "S7 Connection out"=w566:T4)  [unwired: 3 in, 2 out]
        n184 = call-poly <vilib>:"write DB.vi"("Item offset [byte]"=u32 24, "Input STRINGS"=w572, "error in (no error)"=w567, "String length reserved in DB (default=254)"=u16 15, "Data Block #"=w569, "S7 Connection in"=w566) -> ("error out"=w564:errorcluster, "S7 Connection out"=w565:T4)  [unwired: 2 in, 2 out]
        n185 = call-poly <vilib>:"read DB.vi"("error in (no error)"=w564, "items #"=u16 2 ("Items # [byte]"), "Data Block #"=w549, "S7 Connection in"=w565) -> ("error out"=w589:errorcluster, "DINT result array"=w587:i32[], "S7 Connection out"=w584:T4)  [unwired: 5 in]
        n186 = call "PADMINI_AUTO_CYCLE STATE 60.vi"("Enum"=enum16{"Read", "Write"}."Write", "error in (no error)"=w589, "Input"=w587) -> ("error out"=w585:errorcluster)  [unwired: 7 in, 1 out]
        n187 = call-poly <vilib>:"read DB.vi"("Item offset [byte]"=u32 8, "error in (no error)"=w585, "items #"=u16 6 ("Items # [byte]"), "Data Block #"=w549, "S7 Connection in"=w584) -> ("error out"=w577:errorcluster, "REAL result array"=w575:sgl[], "S7 Connection out"=w583:T4)  [unwired: 4 in]
        n188 = call "PADMINI_AUTO_CYCLE VALUE 60.vi"("Enum"=enum16{"Read", "Write"}."Write", "error in (no error)"=w577, "Input"=w575) -> ("error out"=w576:errorcluster)  [unwired: 7 in, 1 out]
        n189 = call-poly <vilib>:"read DB.vi"("Item offset [byte]"=u32 32, "String length reserved in DB (default=254)"=u16 50, "error in (no error)"=w576, "items #"=u16 1 ("Items # [byte]"), "Data Block #"=w549, "S7 Connection in"=w583) -> ("error out"=w554:errorcluster, "STRING result Array"=w551:string[], "S7 Connection out"=w553:T4)  [unwired: 2 in, 1 out]
        n190 = call-poly <vilib>:"read DB.vi"("Item offset [byte]"=u32 84, "String length reserved in DB (default=254)"=u16 10, "error in (no error)"=w554, "items #"=u16 7 ("Items # [byte]"), "Data Block #"=w549, "S7 Connection in"=w553) -> ("error out"=w555:errorcluster, "STRING result Array"=w558:string[], "S7 Connection out"=w552:T4)  [unwired: 2 in, 1 out]
        n191 = Build Array (concatenate)(w551, w558) -> (w550:string[])
        n192 = call "PADMINI_AUTO_BARCODE_STRING 60.vi"("Enum"=enum16{"Read", "Write"}."Write", "error in (no error)"=w555, "Input"=w550) -> ("error out"=w574:errorcluster)  [unwired: 7 in, 1 out]
      }
      frame #1 {
        # "RECONNECT"
        n193 = case shown="Error" w622 {
          selector: w622 -> [w627 w635]
          tunnel: [w626 w632] -> w620
          tunnel: [w627 w633] -> w621
          tunnel: w623 -> [w626 w629]
          tunnel: w619 -> [_ w628]
          frame No Error {
          }
          frame Error {
            n194 = call <vilib>:"Clear Errors.vi"("error in (no error)"=w635) -> ("error out"=w636:errorcluster)  [unwired: 5 in, 1 out]
            n195 = call <vilib>:"disconnect.vi"("error in (no error)"=w636, "S7 Connection in"=w629) -> ("error out"=w634:errorcluster)  [unwired: 8 in, 1 out]
            n196 = call <vilib>:"Clear Errors.vi"("error in (no error)"=w634) -> ("error out"=w631:errorcluster)  [unwired: 5 in, 1 out]
            n197 = call <vilib>:"connect.vi"("PLC Type"=PLC_Type."S7 1200" ("PLC Type 2"), "error in (no error)"=w631, "IP address"=w628) -> ("error out"=w633:errorcluster, "S7 Connection out"=w632:T4)  [unwired: 7 in]
          }
        }
        n198 = Unbundle By Name(w622) -> ("status"=w625:bool)
        n199 = Not(x=w625) -> (.not. x?=w624:bool)
        "PLC 5" <- w624
        n200 = global write "Global 1.vi" "PLC 5"(w624) -> ()
      }
    }
    n201 = call "PADMINI_STOP_ALL.vi"("Enum"=enum16{"Read", "Write"}."Read") -> ("Boolean 2"=w537:bool)  [unwired: 9 in, 1 out]
    n202 = local read "stop"() -> (w536:bool)
    n203 = Or(x=w536, y=w537) -> (x .or. y?=w535:bool)
    n204 = Wait (ms)(milliseconds to wait=u32 50) -> ()  [unwired: 1 out]
  }
  n205 = while {
    shift-right: [w639] -> w101
    shift-left: w21 -> [w649]
    shift-right: [w647] -> w102
    shift-left: w22 -> [w648]
    tunnel: w78 -> [w638]
    stop <- w641 stop-if-true
    # "OP 70 - 80"
    n206 = flat-sequence {
      tunnel: [w660] -> w645
      tunnel: [w708] -> w640
      tunnel: w648 -> [w746]
      tunnel: w649 -> [w745]
      tunnel: w638 -> [w727]
      tunnel: [w727] -> w637
      tunnel: [w799] -> w647
      tunnel: [w798] -> w639
      tunnel: w645 -> [w801]
      tunnel: w640 -> [w800]
      tunnel: w637 -> [w797]
      frame #0 {
        w676 = u16 83 ("Data Block #")
        w701 = u16 81 ("Data Block #")
        w659 = u16 82 ("Data Block #")
        w682 = u16 80 ("Data Block #")
        # "AUTO WRITE"
        n207 = global read "DATA LOG.vi" "OP 70 Outputs"() -> (w744:bool)
        n208 = case shown="True" w744 {
          tunnel: w745 -> [w782 w795]
          tunnel: [w783 w786] -> w706
          tunnel: [w782 w787] -> w705
          tunnel: w746 -> [w783 w792]
          frame False {
          }
          frame True {
            w796 = u16 81  # Data Block #
            n209 = call "PADMINI_AUTO_BARCODE_STATUS 70.vi"("Enum"=enum16{"Read", "Write"}."Read", "error in (no error)"=w792) -> ("error out"=w791:errorcluster, "O/P"=w793:i32[])  [unwired: 8 in]
            n210 = global write "DATA LOG.vi" "OP 70 Outputs"(FALSE) -> ()
            n211 = call-poly <vilib>:"write DB.vi"("DINT input array"=w793, "error in (no error)"=w791, "Data Block #"=w796, "S7 Connection in"=w795) -> ("error out"=w784:errorcluster, "S7 Connection out"=w785:T4)  [unwired: 4 in, 2 out]
            n212 = call-poly <vilib>:"write DB.vi"("DINT input array"=i32[] [0] ("Data Byte"), "error in (no error)"=w784, "Data Block #"=u16 80, "S7 Connection in"=w785) -> ("error out"=w786:errorcluster, "S7 Connection out"=w787:T4)  [unwired: 4 in, 2 out]
          }
        }
        n213 = global read "DATA LOG.vi" "OP 70 reset"() -> (w707:bool)
        n214 = global read "DATA LOG.vi" "Auto Cycle On"() -> (w652:bool)
        n215 = case shown="True" w707 {
          tunnel: w706 -> [w757 w766]
          tunnel: [w757 w765] -> w696
          tunnel: w705 -> [w758 w764]
          tunnel: [w758 w763] -> w697
          frame False {
          }
          frame True {
            n216 = global write "DATA LOG.vi" "OP 70 reset"(FALSE) -> ()
            n217 = call-poly <vilib>:"write DB.vi"("Item offset [byte]"=u16 4 ("Data Block #"), "DINT input array"=i32[] [0], "error in (no error)"=w766, "Data Block #"=u16 80, "S7 Connection in"=w764) -> ("error out"=w765:errorcluster, "S7 Connection out"=w763:T4)  [unwired: 3 in, 2 out]
          }
        }
        n218 = Boolean To (0,1)(Boolean=w652) -> (0, 1=w651:i16)
        n219 = Build Array(w651) -> (w650:i16[])
        n220 = global read "Global 1.vi" "Filtered BARCODE selected"() -> (w698:string[])
        n221 = call-poly <vilib>:"write DB.vi"("Item offset [byte]"=u32 20, "DINT input array"=w650, "error in (no error)"=w696, "Data Block #"=w701, "S7 Connection in"=w697) -> ("error out"=w703:errorcluster, "S7 Connection out"=w704:T4)  [unwired: 3 in, 2 out]
        n222 = call-poly <vilib>:"write DB.vi"("Item offset [byte]"=u32 24, "Input STRINGS"=w698, "error in (no error)"=w703, "String length reserved in DB (default=254)"=u16 15, "Data Block #"=w701, "S7 Connection in"=w704) -> ("error out"=w694:errorcluster, "S7 Connection out"=w695:T4)  [unwired: 2 in, 2 out]
        n223 = call-poly <vilib>:"read DB.vi"("error in (no error)"=w694, "items #"=u16 2 ("Items # [byte]"), "Data Block #"=w682, "S7 Connection in"=w695) -> ("error out"=w742:errorcluster, "DINT result array"=w740:i32[], "S7 Connection out"=w737:T4)  [unwired: 5 in]
        n224 = call "PADMINI_AUTO_CYCLE STATE 70.vi"("Enum"=enum16{"Read", "Write"}."Write", "error in (no error)"=w742, "Input"=w740) -> ("error out"=w738:errorcluster)  [unwired: 7 in, 1 out]
        n225 = call-poly <vilib>:"read DB.vi"("Item offset [byte]"=u32 8, "error in (no error)"=w738, "items #"=u16 2 ("Items # [byte]"), "Data Block #"=w682, "S7 Connection in"=w737) -> ("error out"=w730:errorcluster, "REAL result array"=w728:sgl[], "S7 Connection out"=w736:T4)  [unwired: 4 in]
        n226 = call "PADMINI_AUTO_CYCLE VALUE 70.vi"("Enum"=enum16{"Read", "Write"}."Write", "error in (no error)"=w730, "Input"=w728) -> ("error out"=w729:errorcluster)  [unwired: 7 in, 1 out]
        n227 = call-poly <vilib>:"read DB.vi"("Item offset [byte]"=u32 16, "String length reserved in DB (default=254)"=u16 50, "error in (no error)"=w729, "items #"=u16 1 ("Items # [byte]"), "Data Block #"=w682, "S7 Connection in"=w736) -> ("error out"=w687:errorcluster, "STRING result Array"=w686:string[], "S7 Connection out"=w688:T4)  [unwired: 2 in, 1 out]
        n228 = call-poly <vilib>:"read DB.vi"("Item offset [byte]"=u32 68, "String length reserved in DB (default=254)"=u16 10, "error in (no error)"=w687, "items #"=u16 1 ("Items # [byte]"), "Data Block #"=w682, "S7 Connection in"=w688) -> ("error out"=w689:errorcluster, "STRING result Array"=w690:string[], "S7 Connection out"=w683:T4)  [unwired: 2 in, 1 out]
        n229 = Build Array (concatenate)(w686, w690) -> (w684:string[])
        n230 = call "PADMINI_AUTO_BARCODE_STRING 70.vi"("Enum"=enum16{"Read", "Write"}."Write", "error in (no error)"=w689, "Input"=w684) -> ("error out"=w709:errorcluster)  [unwired: 7 in, 1 out]
        n231 = global read "DATA LOG.vi" "OP 80 Outputs"() -> (w710:bool)
        n232 = case shown="True" w710 {
          tunnel: [w768 w771] -> w681
          tunnel: [w767 w772] -> w657
          tunnel: w709 -> [w768 w778]
          tunnel: w683 -> [w767 w775]
          frame False {
          }
          frame True {
            w781 = u16 83  # Data Block #
            n233 = call "PADMINI_AUTO_BARCODE_STATUS 80.vi"("Enum"=enum16{"Read", "Write"}."Read", "error in (no error)"=w778) -> ("error out"=w777:errorcluster, "O/P"=w779:i32[])  [unwired: 8 in]
            n234 = global write "DATA LOG.vi" "OP 80 Outputs"(FALSE) -> ()
            n235 = call-poly <vilib>:"write DB.vi"("DINT input array"=w779, "error in (no error)"=w777, "Data Block #"=w781, "S7 Connection in"=w775) -> ("error out"=w769:errorcluster, "S7 Connection out"=w770:T4)  [unwired: 4 in, 2 out]
            n236 = call-poly <vilib>:"write DB.vi"("DINT input array"=i32[] [0] ("Data Byte"), "error in (no error)"=w769, "Data Block #"=u16 82, "S7 Connection in"=w770) -> ("error out"=w771:errorcluster, "S7 Connection out"=w772:T4)  [unwired: 4 in, 2 out]
          }
        }
        n237 = global read "DATA LOG.vi" "OP 80 reset"() -> (w680:bool)
        n238 = global read "DATA LOG.vi" "Auto Cycle On"() -> (w655:bool)
        n239 = case shown="True" w680 {
          tunnel: w681 -> [w748 w756]
          tunnel: [w748 w751] -> _
          tunnel: [w748 w751] -> w670
          tunnel: w657 -> [w747 w750]
          tunnel: [w747 w749] -> w656
          frame False {
          }
          frame True {
            n240 = global write "DATA LOG.vi" "OP 80 reset"(FALSE) -> ()
            n241 = call-poly <vilib>:"write DB.vi"("Item offset [byte]"=u16 4 ("Data Block #"), "DINT input array"=i32[] [0], "error in (no error)"=w756, "Data Block #"=u16 82, "S7 Connection in"=w750) -> ("error out"=w751:errorcluster, "S7 Connection out"=w749:T4)  [unwired: 3 in, 2 out]
          }
        }
        n242 = Boolean To (0,1)(Boolean=w655) -> (0, 1=w654:i16)
        n243 = Build Array(w654) -> (w653:i16[])
        n244 = global read "Global 1.vi" "Filtered BARCODE selected"() -> (w673:string[])
        n245 = call-poly <vilib>:"write DB.vi"("Item offset [byte]"=u32 20, "DINT input array"=w653, "error in (no error)"=w670, "Data Block #"=w676, "S7 Connection in"=w656) -> ("error out"=w678:errorcluster, "S7 Connection out"=w679:T4)  [unwired: 3 in, 2 out]
        n246 = call-poly <vilib>:"write DB.vi"("Item offset [byte]"=u32 24, "Input STRINGS"=w673, "error in (no error)"=w678, "String length reserved in DB (default=254)"=u16 15, "Data Block #"=w676, "S7 Connection in"=w679) -> ("error out"=w671:errorcluster, "S7 Connection out"=w672:T4)  [unwired: 2 in, 2 out]
        n247 = call-poly <vilib>:"read DB.vi"("error in (no error)"=w671, "items #"=u16 2 ("Items # [byte]"), "Data Block #"=w659, "S7 Connection in"=w672) -> ("error out"=w712:errorcluster, "DINT result array"=w714:i32[], "S7 Connection out"=w717:T4)  [unwired: 5 in]
        n248 = call "PADMINI_AUTO_CYCLE STATE 80.vi"("Enum"=enum16{"Read", "Write"}."Write", "error in (no error)"=w712, "Input"=w714) -> ("error out"=w716:errorcluster)  [unwired: 7 in, 1 out]
        n249 = call-poly <vilib>:"read DB.vi"("Item offset [byte]"=u32 8, "error in (no error)"=w716, "items #"=u16 1 ("Items # [byte]"), "Data Block #"=w659, "S7 Connection in"=w717) -> ("error out"=w724:errorcluster, "REAL result array"=w726:sgl[], "S7 Connection out"=w718:T4)  [unwired: 4 in]
        n250 = call "PADMINI_AUTO_CYCLE VALUE 80.vi"("Enum"=enum16{"Read", "Write"}."Write", "error in (no error)"=w724, "Input"=w726) -> ("error out"=w725:errorcluster)  [unwired: 7 in, 1 out]
        n251 = call-poly <vilib>:"read DB.vi"("Item offset [byte]"=u32 12, "String length reserved in DB (default=254)"=u16 50, "error in (no error)"=w725, "items #"=u16 1 ("Items # [byte]"), "Data Block #"=w659, "S7 Connection in"=w718) -> ("error out"=w665:errorcluster, "STRING result Array"=w663:string[], "S7 Connection out"=w661:T4)  [unwired: 2 in, 1 out]
        n252 = call-poly <vilib>:"read DB.vi"("Item offset [byte]"=u32 64, "String length reserved in DB (default=254)"=u16 10, "error in (no error)"=w665, "items #"=u16 2 ("Items # [byte]"), "Data Block #"=w659, "S7 Connection in"=w661) -> ("error out"=w664:errorcluster, "STRING result Array"=w669:string[], "S7 Connection out"=w660:T4)  [unwired: 2 in, 1 out]
        n253 = Build Array (concatenate)(w663, w669) -> (w662:string[])
        n254 = call "PADMINI_AUTO_BARCODE_STRING 80.vi"("Enum"=enum16{"Read", "Write"}."Write", "error in (no error)"=w664, "Input"=w662) -> ("error out"=w708:errorcluster)  [unwired: 7 in, 1 out]
      }
      frame #1 {
        # "RECONNECT"
        n255 = case shown="Error" w800 {
          selector: w800 -> [w805 w813]
          tunnel: [w804 w810] -> w798
          tunnel: [w805 w811] -> w799
          tunnel: w801 -> [w804 w807]
          tunnel: w797 -> [_ w806]
          frame No Error {
          }
          frame Error {
            n256 = call <vilib>:"Clear Errors.vi"("error in (no error)"=w813) -> ("error out"=w814:errorcluster)  [unwired: 5 in, 1 out]
            n257 = call <vilib>:"disconnect.vi"("error in (no error)"=w814, "S7 Connection in"=w807) -> ("error out"=w812:errorcluster)  [unwired: 8 in, 1 out]
            n258 = call <vilib>:"Clear Errors.vi"("error in (no error)"=w812) -> ("error out"=w809:errorcluster)  [unwired: 5 in, 1 out]
            n259 = call <vilib>:"connect.vi"("PLC Type"=PLC_Type."S7 1200" ("PLC Type 2"), "error in (no error)"=w809, "IP address"=w806) -> ("error out"=w811:errorcluster, "S7 Connection out"=w810:T4)  [unwired: 7 in]
          }
        }
        n260 = Unbundle By Name(w800) -> ("status"=w803:bool)
        n261 = Not(x=w803) -> (.not. x?=w802:bool)
        "PLC 6" <- w802
        n262 = global write "Global 1.vi" "PLC 6"(w802) -> ()
      }
    }
    n263 = call "PADMINI_STOP_ALL.vi"("Enum"=enum16{"Read", "Write"}."Read") -> ("Boolean 2"=w643:bool)  [unwired: 9 in, 1 out]
    n264 = local read "stop"() -> (w642:bool)
    n265 = Or(x=w642, y=w643) -> (x .or. y?=w641:bool)
    n266 = Wait (ms)(milliseconds to wait=u32 50) -> ()  [unwired: 1 out]
  }
  n267 = while {
    shift-right: [w817] -> w74
    shift-left: w17 -> [w827]
    shift-right: [w825] -> w75
    shift-left: w16 -> [w826]
    tunnel: w77 -> [w816]
    stop <- w819 stop-if-true
    # "OP 90 - 100 - 110"
    n268 = flat-sequence {
      tunnel: [w887] -> w823
      tunnel: [w888] -> w818
      tunnel: w826 -> [w926]
      tunnel: w827 -> [w925]
      tunnel: w816 -> [w907]
      tunnel: [w907] -> w815
      tunnel: [w1016] -> w825
      tunnel: [w1015] -> w817
      tunnel: w823 -> [w1018]
      tunnel: w818 -> [w1017]
      tunnel: w815 -> [w1014]
      frame #0 {
        w853 = u16 72 ("Data Block #")
        w879 = u16 70 ("Data Block #")
        w837 = u16 71 ("Data Block #")
        w867 = u16 69 ("Data Block #")
        # "AUTO WRITE"
        n269 = global read "DATA LOG.vi" "OP 90 Outputs"() -> (w924:bool)
        n270 = case shown="True" w924 {
          tunnel: w925 -> [w999 w1012]
          tunnel: [w1000 w1001] -> w884
          tunnel: [w999 w1002] -> w885
          tunnel: w926 -> [w1000 w1009]
          frame False {
          }
          frame True {
            w1013 = u16 70  # Data Block #
            n271 = call "PADMINI_AUTO_BARCODE_STATUS 90.vi"("Enum"=enum16{"Read", "Write"}."Read", "error in (no error)"=w1009) -> ("error out"=w1008:errorcluster, "O/P"=w1010:i32[])  [unwired: 8 in]
            n272 = global write "DATA LOG.vi" "OP 90 Outputs"(FALSE) -> ()
            n273 = call-poly <vilib>:"write DB.vi"("DINT input array"=w1010, "error in (no error)"=w1008, "Data Block #"=w1013, "S7 Connection in"=w1012) -> ("error out"=w1004:errorcluster, "S7 Connection out"=w1003:T4)  [unwired: 4 in, 2 out]
            n274 = call-poly <vilib>:"write DB.vi"("DINT input array"=i32[] [0] ("Data Byte"), "error in (no error)"=w1004, "Data Block #"=u16 69, "S7 Connection in"=w1003) -> ("error out"=w1001:errorcluster, "S7 Connection out"=w1002:T4)  [unwired: 4 in, 2 out]
          }
        }
        n275 = global read "DATA LOG.vi" "OP 90 reset"() -> (w883:bool)
        n276 = case shown="True" w883 {
          tunnel: w884 -> [w974 w983]
          tunnel: [w974 w982] -> w872
          tunnel: w885 -> [w975 w981]
          tunnel: [w975 w980] -> w873
          frame False {
          }
          frame True {
            n277 = global write "DATA LOG.vi" "OP 90 reset"(FALSE) -> ()
            n278 = call-poly <vilib>:"write DB.vi"("Item offset [byte]"=u16 4 ("Data Block #"), "DINT input array"=i32[] [0], "error in (no error)"=w983, "Data Block #"=u16 69, "S7 Connection in"=w981) -> ("error out"=w982:errorcluster, "S7 Connection out"=w980:T4)  [unwired: 3 in, 2 out]
          }
        }
        n279 = global read "DATA LOG.vi" "Auto Cycle On"() -> (w834:bool)
        n280 = Boolean To (0,1)(Boolean=w834) -> (0, 1=w833:i16)
        n281 = Build Array(w833) -> (w832:i16[])
        n282 = global read "Global 1.vi" "Filtered BARCODE selected"() -> (w882:string[])
        n283 = call-poly <vilib>:"write DB.vi"("Item offset [byte]"=u32 20, "DINT input array"=w832, "error in (no error)"=w872, "Data Block #"=w879, "S7 Connection in"=w873) -> ("error out"=w877:errorcluster, "S7 Connection out"=w876:T4)  [unwired: 3 in, 2 out]
        n284 = call-poly <vilib>:"write DB.vi"("Item offset [byte]"=u32 24, "Input STRINGS"=w882, "error in (no error)"=w877, "String length reserved in DB (default=254)"=u16 15, "Data Block #"=w879, "S7 Connection in"=w876) -> ("error out"=w874:errorcluster, "S7 Connection out"=w875:T4)  [unwired: 2 in, 2 out]
        n285 = call-poly <vilib>:"read DB.vi"("error in (no error)"=w874, "items #"=u16 2 ("Items # [byte]"), "Data Block #"=w867, "S7 Connection in"=w875) -> ("error out"=w922:errorcluster, "DINT result array"=w920:i32[], "S7 Connection out"=w917:T4)  [unwired: 5 in]
        n286 = call "PADMINI_AUTO_CYCLE STATE 90.vi"("Enum"=enum16{"Read", "Write"}."Write", "error in (no error)"=w922, "Input"=w920) -> ("error out"=w918:errorcluster)  [unwired: 7 in, 1 out]
        n287 = call-poly <vilib>:"read DB.vi"("Item offset [byte]"=u32 8, "error in (no error)"=w918, "items #"=u16 2 ("Items # [byte]"), "Data Block #"=w867, "S7 Connection in"=w917) -> ("error out"=w910:errorcluster, "REAL result array"=w908:sgl[], "S7 Connection out"=w916:T4)  [unwired: 4 in]
        n288 = call "PADMINI_AUTO_CYCLE VALUE 90.vi"("Enum"=enum16{"Read", "Write"}."Write", "error in (no error)"=w910, "Input"=w908) -> ("error out"=w909:errorcluster)  [unwired: 7 in, 1 out]
        n289 = call-poly <vilib>:"read DB.vi"("Item offset [byte]"=u32 16, "String length reserved in DB (default=254)"=u16 50, "error in (no error)"=w909, "items #"=u16 1 ("Items # [byte]"), "Data Block #"=w867, "S7 Connection in"=w916) -> ("error out"=w871:errorcluster, "STRING result Array"=w862:string[], "S7 Connection out"=w870:T4)  [unwired: 2 in, 1 out]
        n290 = call-poly <vilib>:"read DB.vi"("Item offset [byte]"=u32 68, "String length reserved in DB (default=254)"=u16 10, "error in (no error)"=w871, "items #"=u16 3 ("Items # [byte]"), "Data Block #"=w867, "S7 Connection in"=w870) -> ("error out"=w869:errorcluster, "STRING result Array"=w861:string[], "S7 Connection out"=w868:T4)  [unwired: 2 in, 1 out]
        n291 = Build Array (concatenate)(w862, w861) -> (w860:string[])
        n292 = call "PADMINI_AUTO_BARCODE_STRING 90.vi"("Enum"=enum16{"Read", "Write"}."Write", "error in (no error)"=w869, "Input"=w860) -> ("error out"=w889:errorcluster)  [unwired: 7 in, 1 out]
        n293 = global read "DATA LOG.vi" "OP 100 Outputs"() -> (w890:bool)
        n294 = case shown="True" w890 {
          tunnel: w868 -> [w984 w997]
          tunnel: [w985 w988] -> w858
          tunnel: [w984 w989] -> w859
          tunnel: w889 -> [w985 w994]
          frame False {
          }
          frame True {
            w998 = u16 72  # Data Block #
            n295 = call "PADMINI_AUTO_BARCODE_STATUS 100.vi"("Enum"=enum16{"Read", "Write"}."Read", "error in (no error)"=w994) -> ("error out"=w993:errorcluster, "O/P"=w995:i32[])  [unwired: 8 in]
            n296 = global write "DATA LOG.vi" "OP 100 Outputs"(FALSE) -> ()
            n297 = call-poly <vilib>:"write DB.vi"("DINT input array"=w995, "error in (no error)"=w993, "Data Block #"=w998, "S7 Connection in"=w997) -> ("error out"=w987:errorcluster, "S7 Connection out"=w986:T4)  [unwired: 4 in, 2 out]
            n298 = call-poly <vilib>:"write DB.vi"("DINT input array"=i32[] [0] ("Data Byte"), "error in (no error)"=w987, "Data Block #"=u16 71, "S7 Connection in"=w986) -> ("error out"=w988:errorcluster, "S7 Connection out"=w989:T4)  [unwired: 4 in, 2 out]
          }
        }
        n299 = global read "DATA LOG.vi" "OP 100 reset"() -> (w857:bool)
        n300 = case shown="True" w857 {
          tunnel: w858 -> [w964 w973]
          tunnel: [w964 w972] -> w849
          tunnel: w859 -> [w965 w971]
          tunnel: [w965 w970] -> w848
          frame False {
          }
          frame True {
            n301 = global write "DATA LOG.vi" "OP 100 reset"(FALSE) -> ()
            n302 = call-poly <vilib>:"write DB.vi"("Item offset [byte]"=u16 4 ("Data Block #"), "DINT input array"=i32[] [0], "error in (no error)"=w973, "Data Block #"=u16 71, "S7 Connection in"=w971) -> ("error out"=w972:errorcluster, "S7 Connection out"=w970:T4)  [unwired: 3 in, 2 out]
          }
        }
        n303 = global read "DATA LOG.vi" "Auto Cycle On"() -> (w831:bool)
        n304 = Boolean To (0,1)(Boolean=w831) -> (0, 1=w830:i16)
        n305 = Build Array(w830) -> (w829:i16[])
        n306 = global read "Global 1.vi" "Filtered BARCODE selected"() -> (w850:string[])
        n307 = call-poly <vilib>:"write DB.vi"("Item offset [byte]"=u32 20, "DINT input array"=w829, "error in (no error)"=w849, "Data Block #"=w853, "S7 Connection in"=w848) -> ("error out"=w855:errorcluster, "S7 Connection out"=w856:T4)  [unwired: 3 in, 2 out]
        n308 = call-poly <vilib>:"write DB.vi"("Item offset [byte]"=u32 24, "Input STRINGS"=w850, "error in (no error)"=w855, "String length reserved in DB (default=254)"=u16 15, "Data Block #"=w853, "S7 Connection in"=w856) -> ("error out"=w846:errorcluster, "S7 Connection out"=w847:T4)  [unwired: 2 in, 2 out]
        n309 = call-poly <vilib>:"read DB.vi"("error in (no error)"=w846, "items #"=u16 2 ("Items # [byte]"), "Data Block #"=w837, "S7 Connection in"=w847) -> ("error out"=w892:errorcluster, "DINT result array"=w894:i32[], "S7 Connection out"=w897:T4)  [unwired: 5 in]
        n310 = call "PADMINI_AUTO_CYCLE STATE 100.vi"("Enum"=enum16{"Read", "Write"}."Write", "error in (no error)"=w892, "Input"=w894) -> ("error out"=w896:errorcluster)  [unwired: 7 in, 1 out]
        n311 = call-poly <vilib>:"read DB.vi"("Item offset [byte]"=u32 8, "error in (no error)"=w896, "items #"=u16 11 ("Items # [byte]"), "Data Block #"=w837, "S7 Connection in"=w897) -> ("error out"=w904:errorcluster, "REAL result array"=w906:sgl[], "S7 Connection out"=w898:T4)  [unwired: 4 in]
        n312 = call "PADMINI_AUTO_CYCLE VALUE 100.vi"("Enum"=enum16{"Read", "Write"}."Write", "error in (no error)"=w904, "Input"=w906) -> ("error out"=w905:errorcluster)  [unwired: 7 in, 1 out]
        n313 = call-poly <vilib>:"read DB.vi"("Item offset [byte]"=u32 52, "String length reserved in DB (default=254)"=u16 50, "error in (no error)"=w905, "items #"=u16 1 ("Items # [byte]"), "Data Block #"=w837, "S7 Connection in"=w898) -> ("error out"=w843:errorcluster, "STRING result Array"=w840:string[], "S7 Connection out"=w842:T4)  [unwired: 2 in, 1 out]
        n314 = call-poly <vilib>:"read DB.vi"("Item offset [byte]"=u32 104, "String length reserved in DB (default=254)"=u16 10, "error in (no error)"=w843, "items #"=u16 2 ("Items # [byte]"), "Data Block #"=w837, "S7 Connection in"=w842) -> ("error out"=w844:errorcluster, "STRING result Array"=w838:string[], "S7 Connection out"=w841:T4)  [unwired: 2 in, 1 out]
        n315 = Build Array (concatenate)(w840, w838) -> (w839:string[])
        n316 = call "PADMINI_AUTO_BARCODE_STRING 100.vi"("Enum"=enum16{"Read", "Write"}."Write", "error in (no error)"=w844, "Input"=w839) -> ("error out"=w886:errorcluster)  [unwired: 7 in, 1 out]
        n317 = disable-structure shown="Enabled" {
          disable-tunnel: [w946 w962] -> w888
          disable-tunnel: [w945 w963] -> w887
          disable-tunnel: w886 -> [w944 w962]
          disable-tunnel: w841 -> [w943 w963]
          frame Disabled {
            w936 = u16 75 ("Data Block #")
            # "OP100 OK\nOP 100 NG"
            n318 = global read "DATA LOG.vi" "OP 110 Outputs"() -> (w942:bool)
            n319 = case shown="True" w942 {
              tunnel: [w947 w952] -> w928
              tunnel: [w948 w953] -> w929
              tunnel: w944 -> [w947 w957]
              tunnel: w943 -> [w948 w956]
              frame False {
              }
              frame True {
                w949 = i32[] [0]  # DINT input array
                w950 = u16 75  # Data Block #
                n320 = call "PADMINI_AUTO_BARCODE_STATUS 110.vi"("Enum"=enum16{"Read", "Write"}."Read", "error in (no error)"=w957) -> ("error out"=w959:errorcluster, "O/P"=w960:i32[])  [unwired: 8 in]
                n321 = call-poly <vilib>:"write DB.vi"("Item offset [byte]"=u32 4, "DINT input array"=w960, "error in (no error)"=w959, "Data Block #"=w950, "S7 Connection in"=w956) -> ("error out"=w951:errorcluster, "S7 Connection out"=w954:T4)  [unwired: 3 in, 2 out]
                n322 = global write "DATA LOG.vi" "OP 110 Outputs"(FALSE) -> ()
                n323 = call-poly <vilib>:"write DB.vi"("DINT input array"=w949, "error in (no error)"=w951, "Data Block #"=w950, "S7 Connection in"=w954) -> ("error out"=w952:errorcluster, "S7 Connection out"=w953:T4)  [unwired: 4 in, 2 out]
              }
            }
            n324 = call-poly <vilib>:"read DB.vi"("error in (no error)"=w928, "items #"=u16 1 ("Items # [byte]"), "Data Block #"=w936, "S7 Connection in"=w929) -> ("error out"=w940:errorcluster, "DINT result array"=w938:i32[], "S7 Connection out"=w937:T4)  [unwired: 5 in]
            n325 = call "PADMINI_AUTO_CYCLE STATE 110.vi"("Enum"=enum16{"Read", "Write"}."Write", "error in (no error)"=w940, "Input"=w938) -> ("error out"=w930:errorcluster)  [unwired: 7 in, 1 out]
            n326 = call-poly <vilib>:"read DB.vi"("Item offset [byte]"=u32 12, "String length reserved in DB (default=254)"=u16 50, "error in (no error)"=w930, "items #"=u16 1 ("Items # [byte]"), "Data Block #"=w936, "S7 Connection in"=w937) -> ("error out"=w932:errorcluster, "STRING result Array"=w933:string[], "S7 Connection out"=w945:T4)  [unwired: 2 in, 1 out]
            n327 = call "PADMINI_AUTO_BARCODE_STRING 110.vi"("Enum"=enum16{"Read", "Write"}."Write", "error in (no error)"=w932, "Input"=w933) -> ("error out"=w946:errorcluster)  [unwired: 7 in, 1 out]
          }
          frame Enabled {
          }
        }
      }
      frame #1 {
        # "RECONNECT"
        n328 = case shown="Error" w1017 {
          selector: w1017 -> [w1022 w1030]
          tunnel: [w1021 w1027] -> w1015
          tunnel: [w1022 w1028] -> w1016
          tunnel: w1018 -> [w1021 w1024]
          tunnel: w1014 -> [_ w1023]
          frame No Error {
          }
          frame Error {
            n329 = call <vilib>:"Clear Errors.vi"("error in (no error)"=w1030) -> ("error out"=w1031:errorcluster)  [unwired: 5 in, 1 out]
            n330 = call <vilib>:"disconnect.vi"("error in (no error)"=w1031, "S7 Connection in"=w1024) -> ("error out"=w1029:errorcluster)  [unwired: 8 in, 1 out]
            n331 = call <vilib>:"Clear Errors.vi"("error in (no error)"=w1029) -> ("error out"=w1026:errorcluster)  [unwired: 5 in, 1 out]
            n332 = call <vilib>:"connect.vi"("PLC Type"=PLC_Type."S7 1200" ("PLC Type 2"), "error in (no error)"=w1026, "IP address"=w1023) -> ("error out"=w1028:errorcluster, "S7 Connection out"=w1027:T4)  [unwired: 7 in]
          }
        }
        n333 = Unbundle By Name(w1017) -> ("status"=w1020:bool)
        n334 = Not(x=w1020) -> (.not. x?=w1019:bool)
        "PLC 7" <- w1019
        n335 = global write "Global 1.vi" "PLC 7"(w1019) -> ()
      }
    }
    n336 = call "PADMINI_STOP_ALL.vi"("Enum"=enum16{"Read", "Write"}."Read") -> ("Boolean 2"=w821:bool)  [unwired: 9 in, 1 out]
    n337 = local read "stop"() -> (w820:bool)
    n338 = Or(x=w820, y=w821) -> (x .or. y?=w819:bool)
    n339 = Wait (ms)(milliseconds to wait=u32 50) -> ()  [unwired: 1 out]
  }
  n340 = while {
    shift-right: [w1034] -> w2
    shift-left: w12 -> [w1044]
    shift-right: [w1042] -> w3
    shift-left: w13 -> [w1043]
    tunnel: w5 -> [w1033]
    stop <- w1036 stop-if-true
    # "OP 110"
    n341 = flat-sequence {
      tunnel: [w1063] -> w1040
      tunnel: [w1064] -> w1035
      tunnel: w1043 -> [w1067]
      tunnel: w1044 -> [w1066]
      tunnel: w1033 -> [w1065]
      tunnel: [w1065] -> w1032
      tunnel: [w1096] -> w1042
      tunnel: [w1095] -> w1034
      tunnel: w1040 -> [w1098]
      tunnel: w1035 -> [w1097]
      tunnel: w1032 -> [w1094]
      frame #0 {
        w1054 = u16 7 ("Data Block #")
        # "OP100 OK\nOP 100 NG"
        # "AUTO WRITE"
        n342 = disable-structure shown="Enabled" {
          disable-tunnel: w1067 -> [w1076 w1077]
          disable-tunnel: w1066 -> [w1075 w1078]
          disable-tunnel: [w1074 w1078] -> w1062
          disable-tunnel: [w1073 w1077] -> w1061
          frame Disabled {
            n343 = global read "DATA LOG.vi" "Auto Cycle On"() -> (w1070:bool)
            n344 = Boolean To (0,1)(Boolean=w1070) -> (0, 1=w1069:i16)
            n345 = Build Array(w1069) -> (w1068:i16[])
            n346 = call-poly <vilib>:"write DB.vi"("Item offset [byte]"=u32 20, "DINT input array"=w1068, "error in (no error)"=w1076, "Data Block #"=u16 72, "S7 Connection in"=w1075) -> ("error out"=w1073:errorcluster, "S7 Connection out"=w1074:T4)  [unwired: 3 in, 2 out]
          }
          frame Enabled {
          }
        }
        n347 = global read "DATA LOG.vi" "OP 110 Outputs"() -> (w1060:bool)
        n348 = case shown="True" w1060 {
          tunnel: [w1079 w1084] -> w1047
          tunnel: [w1080 w1085] -> w1048
          tunnel: w1061 -> [w1079 w1089]
          tunnel: w1062 -> [w1080 w1088]
          frame False {
          }
          frame True {
            w1081 = i32[] [0]  # DINT input array
            w1082 = u16 7  # Data Block #
            n349 = call "PADMINI_AUTO_BARCODE_STATUS 110.vi"("Enum"=enum16{"Read", "Write"}."Read", "error in (no error)"=w1089) -> ("error out"=w1091:errorcluster, "O/P"=w1092:i32[])  [unwired: 8 in]
            n350 = call-poly <vilib>:"write DB.vi"("Item offset [byte]"=u32 4, "DINT input array"=w1092, "error in (no error)"=w1091, "Data Block #"=w1082, "S7 Connection in"=w1088) -> ("error out"=w1083:errorcluster, "S7 Connection out"=w1086:T4)  [unwired: 3 in, 2 out]
            n351 = global write "DATA LOG.vi" "OP 110 Outputs"(FALSE) -> ()
            n352 = call-poly <vilib>:"write DB.vi"("DINT input array"=w1081, "error in (no error)"=w1083, "Data Block #"=w1082, "S7 Connection in"=w1086) -> ("error out"=w1084:errorcluster, "S7 Connection out"=w1085:T4)  [unwired: 4 in, 2 out]
          }
        }
        n353 = call-poly <vilib>:"read DB.vi"("error in (no error)"=w1047, "items #"=u16 1 ("Items # [byte]"), "Data Block #"=w1054, "S7 Connection in"=w1048) -> ("error out"=w1058:errorcluster, "DINT result array"=w1056:i32[], "S7 Connection out"=w1055:T4)  [unwired: 5 in]
        n354 = call "PADMINI_AUTO_CYCLE STATE 110.vi"("Enum"=enum16{"Read", "Write"}."Write", "error in (no error)"=w1058, "Input"=w1056) -> ("error out"=w1045:errorcluster)  [unwired: 7 in, 1 out]
        "error out 3" <- w1045
        n355 = call-poly <vilib>:"read DB.vi"("Item offset [byte]"=u32 12, "String length reserved in DB (default=254)"=u16 50, "error in (no error)"=w1045, "items #"=u16 3 ("Items # [byte]"), "Data Block #"=w1054, "S7 Connection in"=w1055) -> ("error out"=w1050:errorcluster, "STRING result Array"=w1051:string[], "S7 Connection out"=w1063:T4)  [unwired: 2 in, 1 out]
        n356 = call "PADMINI_AUTO_BARCODE_STRING 110.vi"("Enum"=enum16{"Read", "Write"}."Write", "error in (no error)"=w1050, "Input"=w1051) -> ("error out"=w1064:errorcluster)  [unwired: 7 in, 1 out]
        "error out 2" <- w1064
      }
      frame #1 {
        # "RECONNECT"
        n357 = case shown="Error" w1097 {
          selector: w1097 -> [w1102 w1110]
          tunnel: [w1101 w1107] -> w1095
          tunnel: [w1102 w1108] -> w1096
          tunnel: w1098 -> [w1101 w1104]
          tunnel: w1094 -> [_ w1103]
          frame No Error {
          }
          frame Error {
            n358 = call <vilib>:"Clear Errors.vi"("error in (no error)"=w1110) -> ("error out"=w1111:errorcluster)  [unwired: 5 in, 1 out]
            n359 = call <vilib>:"disconnect.vi"("error in (no error)"=w1111, "S7 Connection in"=w1104) -> ("error out"=w1109:errorcluster)  [unwired: 8 in, 1 out]
            n360 = call <vilib>:"Clear Errors.vi"("error in (no error)"=w1109) -> ("error out"=w1106:errorcluster)  [unwired: 5 in, 1 out]
            n361 = call <vilib>:"connect.vi"("PLC Type"=PLC_Type."S7 1200" ("PLC Type 2"), "error in (no error)"=w1106, "IP address"=w1103) -> ("error out"=w1108:errorcluster, "S7 Connection out"=w1107:T4)  [unwired: 7 in]
          }
        }
        n362 = Unbundle By Name(w1097) -> ("status"=w1100:bool)
        n363 = Not(x=w1100) -> (.not. x?=w1099:bool)
        "PLC 8" <- w1099
        n364 = global write "Global 1.vi" "PLC 8"(w1099) -> ()
      }
    }
    n365 = call "PADMINI_STOP_ALL.vi"("Enum"=enum16{"Read", "Write"}."Read") -> ("Boolean 2"=w1038:bool)  [unwired: 9 in, 1 out]
    n366 = local read "stop"() -> (w1037:bool)
    n367 = Or(x=w1037, y=w1038) -> (x .or. y?=w1036:bool)
    n368 = Wait (ms)(milliseconds to wait=u32 50) -> ()  [unwired: 1 out]
  }
  n369 = call <vilib>:"Clear Errors.vi"("error in (no error)"=w3) -> ("error out"=w4:errorcluster)  [unwired: 5 in, 1 out]
  n370 = call <vilib>:"disconnect.vi"("error in (no error)"=w4, "S7 Connection in"=w2) -> ("error out"=w1:errorcluster)  [unwired: 8 in, 1 out]
  n371 = call <vilib>:"Clear Errors.vi"("error in (no error)"=w151) -> ("error out"=w152:errorcluster)  [unwired: 5 in, 1 out]
  n372 = call <vilib>:"Clear Errors.vi"("error in (no error)"=w158) -> ("error out"=w160:errorcluster)  [unwired: 5 in, 1 out]
  n373 = call <vilib>:"Clear Errors.vi"("error in (no error)"=w120) -> ("error out"=w121:errorcluster)  [unwired: 5 in, 1 out]
  n374 = call <vilib>:"Clear Errors.vi"("error in (no error)"=w137) -> ("error out"=w136:errorcluster)  [unwired: 5 in, 1 out]
  n375 = call <vilib>:"disconnect.vi"("error in (no error)"=w121, "S7 Connection in"=w119) -> ("error out"=w116:errorcluster)  [unwired: 8 in, 1 out]
  n376 = call <vilib>:"Clear Errors.vi"("error in (no error)"=w102) -> ("error out"=w103:errorcluster)  [unwired: 5 in, 1 out]
  n377 = call <vilib>:"disconnect.vi"("error in (no error)"=w103, "S7 Connection in"=w101) -> ("error out"=w73:errorcluster)  [unwired: 8 in, 1 out]
  n378 = call <vilib>:"disconnect.vi"("error in (no error)"=w136, "S7 Connection in"=w138) -> ("error out"=w117:errorcluster)  [unwired: 8 in, 1 out]
  n379 = call <vilib>:"disconnect.vi"("error in (no error)"=w160, "S7 Connection in"=w159) -> ("error out"=w148:errorcluster)  [unwired: 8 in, 1 out]
  n380 = call <vilib>:"disconnect.vi"("error in (no error)"=w152, "S7 Connection in"=w150) -> ("error out"=w149:errorcluster)  [unwired: 8 in, 1 out]
  n381 = call <vilib>:"Clear Errors.vi"("error in (no error)"=w75) -> ("error out"=w76:errorcluster)  [unwired: 5 in, 1 out]
  n382 = Merge Errors(w148, w149, w117, w116) -> (w147:errorcluster)
  n383 = call <vilib>:"Clear Errors.vi"("error in (no error)"=w197) -> ("error out"=w185:errorcluster)  [unwired: 5 in, 1 out]
  n384 = call <vilib>:"disconnect.vi"("error in (no error)"=w76, "S7 Connection in"=w74) -> ("error out"=w71:errorcluster)  [unwired: 8 in, 1 out]
  n385 = call <vilib>:"disconnect.vi"("error in (no error)"=w185, "S7 Connection in"=w184) -> ("error out"=w183:errorcluster)  [unwired: 8 in, 1 out]
  n386 = Merge Errors(w73, w71, w1) -> (w72:errorcluster)
  n387 = Merge Errors(w183, w147, w72) -> (w202:errorcluster)
  n388 = call <vilib>:"Simple Error Handler.vi"("type of dialog (OK msg:1)"=w53, "error in (no error)"=w202) -> ("error out"=w201:errorcluster)  [unwired: 3 in, 4 out]
  n389 = control-ref of="This VI"() -> (w54:refnum<vi>)
  n390 = call <vilib>:"Clear Errors.vi"("error in (no error)"=w201) -> ("error out"=w200:errorcluster)  [unwired: 5 in, 1 out]
  n391 = invoke class="VI" method="FP.Close"(reference=w54, error in=w200) -> (error out=→"error out":errorcluster)  [unwired: 1 in, 2 out]
